vi "QuantelDataGrabSERI.vi"(9 "stop":bool) -> ()   [LabVIEW 2022 SP3]
uses:
  ScanningControl/Motion Controllers/-MotionRoutines/MotionGlobals.vi
  ScanningControl/Motion Controllers/NI_controller/-NI_MotionRoutines/MotionSys.ctl
  ScanningControl/-ScanSystem/Controls/location.ctl
  <instrlib>/Acqiris Bx/Acqiris Bx.lvlib
  <instrlib>/LeCroy Wave Series/LeCroy Wave Series.lvlib
  <vilib>/ptbypt/NI_PtbyPt.lvlib
  <vilib>/picture/picture.llb/imagedata.ctl
  <vilib>/Utility/miscctls.llb/LVRectTypeDef.ctl
  <vilib>/Utility/miscctls.llb/LVBoundsTypeDef.ctl
  <instrlib>/Acqiris Dx/Acqiris Dx.lvlib
  ScanningControl/Digitizers/-DigitizerRoutines/Digitizer.ctl
  ScanningControl/Motion Controllers/-MotionRoutines/ScanAxis.ctl
  ScanningControl/Motion Controllers/NI_controller/-NI_MotionRoutines/MotionParameters.ctl
  Patient Routines/PatientGlobals.vi
  ScanningControl/Digitizers/-DigitizerRoutines/DigitizerGlobals.vi
  ScanningControl/Motion Controllers/-MotionRoutines/3rdAxis.ctl
  <vilib>/DAQmx/write.llb/DAQmx Write (Digital Bool 1Line 1Point).vi
panel:
  in  "Overide Gain?":bool
  in  "Sector?":bool=TRUE
  in  "Fill\nSpace":bool
  out "File Name":string="none"
  in  "1:1\nAspect":bool
  out "append letter":i8=65
  in  "Visible":bool
  in  "Center":bool
  in  "c (m/s)":dbl=1485.0
  in  "Tab Control":enum32{"Acquire", "Custom Settings"}(tab)
  in  "Gain":dbl(ring)=0.2 items=["7"=8.0, "6"=4.0, "5"=2.0, "4"=0.8, "3"=0.4, "2"=0.2, "1"=0.08]
  in  "View Queue":bool
  out "No data\nEntering\nQueue":bool
  in  "Probe":u16(ring) items=["Aviso Sector 10 MHz", "Aviso Sector 20 MHz Retina", "Aviso Sector 20 MHz", "Aviso Lin50", "Custom"]
  out "fps":dbl format="%#.2g"
  in  "Save All Queue":bool
  in  "Flush Queue":bool
  in  "Pause":bool=TRUE
  out "In Queue":u8 max=50 step=1
  in  "Plane":i8(knob) min=0 max=12 step=3 scale=0.0..12.0
  in  "Patient Info":bool
  out "queue bar":u8(slide) scale=0.0..100.0
  in  "Scan Location":enum32{"Radio Selection 1", "Radio Selection 2"}(radio)
  in  "Save Raw":bool
  in  "SetDig":bool
  in  "Gate Length":dbl=0.15 format="%.6f"
  in  "LowTime":dbl=0.0001
  in  "Acquisition Parameters":T1={"Sampling Rate"=250.0, "Ref Delay (ms)"=0.0, "rf points per line"=2048, "rf lines"=256, "Dig Scale"=4.0} {"Dig Scale" items=["8 V"=8.0, "4 V"=4.0, "2 V"=2.0, "800 mV"=0.8, "400 mV"=0.4, "200 mV"=0.2, "80 mV"=0.08]; "rf lines" min=1; "rf points per line" min=1; "Ref Delay (ms)" format="%.2f"}
  in  "Filter Prams":T2={"low cutoff"=20, "order"=81, "high cutoff"=60}
  in  "Type of Mean":u16(ring)=4 items=["Mean from lines", "Mean just lines", "Poly Mean", "No mean", "Filter"]
  in  "distance?":bool=TRUE
  in  "Scan Info":T3
  in  "Timeout (s)":dbl=0.05
  in  "Software Gate":bool=TRUE
  in  "Bang Trig":bool=TRUE
  in  "N to save":u8=100 min=1 max=100 step=1
  out "Current Image":i32
  in  "Save Setting Profile":bool=TRUE
  in  "dB Range":cluster{i32, i32}(slide)={-65, 0}
  out "Raw data":dbl[][](graph)
  # "dB"
  # "Ruler"
  # "Do not adjust!!!!!"
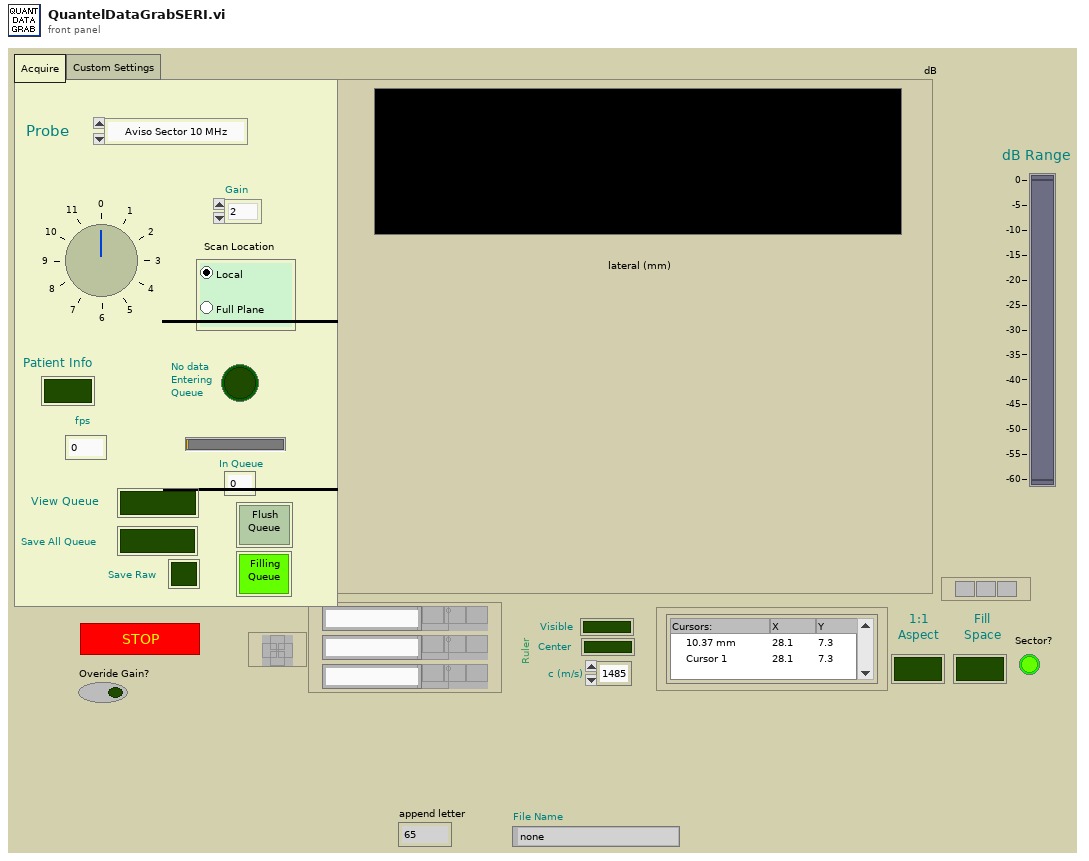
[diagram p1: front panel]
types:
  T1 = cluster{"Sampling Rate":dbl, "Ref Delay (ms)":dbl, "rf points per line":i32, "rf lines":i32, "Dig Scale":dbl}
  T2 = cluster{"low cutoff":i32, "order":i32, "high cutoff":i32}
  T3 = cluster{"delay":sgl, "pivot distance":sgl, "sector scan angle":sgl, "operator":string, "Scan Mode":string, "location":string}
  T4 = typedef "MotionParameters.ctl" = cluster{"No Motion?":bool, "Motion System":T5, "Motion Bd ID":u8, "Motion Profile":string, "# Axis":i8, "Reverse Z axis?":bool, "SMAC Axis":u16, "scan pair":T6, "RT fps":sgl, "Steps per mm":i32[], "Motor Parameters":cluster{"velocity ct/s":dbl[], "accel ct/s^2":dbl[]}, "One Way Scan":bool, "Reverse One Way Scan":bool, "Global Position (mm)":dbl[], "Plane":i32, "Distance between\nscan lines (um)":sgl, "Distance between\nscan planes (um)":sgl, "number of scan planes":i32, "Total steps in line":i32, "Xtra plane\ndistance  (um)":i32, "Xtra planes ":i32, "Add Axis":bool, "overshoot cts":i32, "BKPT Shift":i32, "Scan Start Time (ms)":u32, "ESP VISA":refnum<visa-resource-name>, "3rd Axis":T7, "GL Ref Out":refnum<k7>, "Galil Address":string}
  T5 = typedef "MotionSys.ctl" = enum16{"MM3000", "NI 735x", "Newport ESP", "No Motion Card", "Galil"}
  T6 = typedef "ScanAxis.ctl" = enum16{"y-(x) scan", "x-(y) scan", "z-(x) scan", "z-(y) scan", "y-(z) scan", "x-(z) scan", "w-(x) scan", "w-(y) scan", "w-(z) scan", "x-(w) scan", "y-(w) scan", "z-(w) scan"}
  T7 = typedef "3rdAxis.ctl" = u16
  T8 = typedef "LVBoundsTypeDef.ctl" = cluster{"Width":u32, "Height":u32}
  T9 = typedef "LVRectTypeDef.ctl" = cluster{"Left":i16, "Top":i16, "Right":i16, "Bottom":i16}
  T10 = typedef "Digitizer.ctl" = enum16{"Acqiris Digitizer", "NI Digitizer", "LeCroy", "GaGe", "AlazarTech", "No Digitizer", "Teledyne"}
  T11 = cluster{"gain":dbl, bool, "wfm":i16[][], "max queue size (-1, unlimited)":i32, bool}
  T12 = cluster{"DataBufferQ":refnum<queue>, "LastNQ":refnum<queue>, "LastN_JPG_Q":refnum<queue>, "Stop":refnum<notifier>}
  T13 = typedef "imagedata.ctl" = cluster{"image type":i32, "image depth":i32, "image":u8[], "mask":u8[], "colors":u32[], "Rectangle":cluster{"left":i16, "top":i16, "right":i16, "bottom":i16}}
  T14 = typedef "location.ctl" = enum16{"Automatic", "WCM Main", "Hawaii", "Columbia MM3000", "Columbia  NI System", "NYU", "RRI 2", "UHI Allen", "CUMC RT", "Chiba", "Stony Brook", "WCM Microscopy", "WCM Aeoretch", "WCM Optics Lab", "WCM Main 2Axis", "WCM Rotation", "WCM SAM SMAC", "SERI GP"}
  T15 = cluster{"Voltage Scale":dbl, "Offset":dbl, "Coupling":u16}
  T16 = cluster{"Source":u16, "Coupling":u16, "Slope":u16, "Level":dbl}
  T17 = cluster{"Source":u16, "Coupling":u16, "Slope":u16, "Level (mV)":dbl}
  T18 = cluster{"DataBufferQ":refnum<queue>, "LastNQ":refnum<queue>, "LastNBMPQ":refnum<queue>, "SaveRawN":refnum<notifier>, "StopN":refnum<notifier>}
  T19 = cluster{"NI Dig":refnum<k15>, "Lecroy":refnum<visa-resource-name>, "Alazar":i32, "Acqiris":string}
  T20 = typedef "DigitizerSettings.ctl" = cluster{"Digitizer delay (us) ":dbl, "rf points per line":i32, "lines per plane":i32, "Samp Rate (Hz)":dbl, "Additional dig delay (us)":dbl, "Voltage Scale":dbl, "Pre-Looks":i32, "Offset delay (us)":dbl, "bits A/D":i8, "Avg Num":i32, "DigTimeOut":sgl, "Rel Dig Delay":sgl, "Dig Ch":i32, "LeCroyCluster":cluster{"LeCroy Channels":bool[], "LC read pt offset":dbl, "Sweep Avg":bool}, "Main Digitizer":T10, "Dig Config":T21, "Digitizer ID Cluster":T22, "Trigger Settings":cluster{"Trig Source":u16, "Trig Coupling":u16, "Trig Slope":u16, "Level (mV)":dbl}, "Bulk Acq":bool, "Bulk Start Indexes":i32[], "Data Ref RF":refnum<data-value>, "NI ID/Channel":cluster{"NI ID":refnum<k15>, "NI CH":i32}[], "Total Dig CH":i32, "Xtra Ann Trig delay (us)":dbl, "Fix Z Delay?":bool, "One Way Transmission?":bool, "Data Ref Log":refnum<data-value>}
  T21 = typedef "DigConfig.ctl" = enum16{"Single channel", "2 Chans w/ 2 Acqiris", "2 Chans w/ 1 Acqiris", "5-CH Pulser New", "5-CH pulser w/ ann array", "5-pass style ann array", "Empty"}
  T22 = typedef "DigitizerID.ctl" = cluster{"Acqiris/Alazar/SP ID":u32[], "NI Instr Handles":refnum<k15>[], "LeCroy VISA":refnum<visa-resource-name>, "GaGe Handle":cluster{"Handle":u32, "Sample size":u32, "Resolution":i32, "Offset":i32, "Channels":u32, "Boards":u32}, "ATS Ref":string, "Acqiris Address":string[], "ADQRef":refnum<k24>, "adq_cu_ptr":refnum<k24>}
  T23 = cluster{"Handle":u32, "Sample size":u32, "Resolution":i32, "Offset":i32, "Channels":u32, "Boards":u32}
  T24 = typedef "LVStringsAndValuesArrayTypeDef_DBL.ctl" = cluster{"String":string, "Value":dbl}[]
  T25 = cluster{"Case name":string, "Distance between\nscan lines (mm)":sgl, "Acquistion Parameters":cluster{"Sampling Rate":dbl, "Ref Delay (ms)":dbl, "rf points per line":i32, "rf lines":i32, "Dig Scale":dbl}, "Timeout (s)":dbl, "Sector?":bool, "Filter Prams":cluster{"low cutoff":i32, "order":i32, "high cutoff":i32}, "Scan Info":cluster{"delay":sgl, "pivot distance":sgl, "sector scan angle":sgl, "operator":string, "Scan Mode":string, "location":string}}[]
  T26 = cluster{"Case name":string, "Distance between\nscan lines (mm)":sgl, "Acquistion Parameters":cluster{"Sampling Rate":dbl, "Ref Delay (ms)":dbl, "rf points per line":i32, "rf lines":i32, "Dig Scale":dbl}, "Timeout (s)":dbl, "Sector?":bool, "Filter Prams":cluster{"low cutoff":i32, "order":i32, "high cutoff":i32}, "Scan Info":cluster{"delay":sgl, "pivot distance":sgl, "sector scan angle":sgl, "operator":string, "Scan Mode":string, "location":string}}
  T27 = cluster{"Y Scale Offset":dbl, "Y Scale Multi":dbl, "X Scale Offset":dbl, "X Scale Multi":dbl, "Gate Distance":dbl}
  T28 = cluster{"data value reference":refnum<data-value>, "bytes to transfer":u32, "rf pts actual":u32}
  T29 = cluster{"Axis scaling Params":cluster{"X right":dbl, "X left":dbl, "Y low":dbl, "Y high":dbl}, "x scaled":dbl[][], "y scaled":dbl[][], "scales":cluster{"inc x (mm)":dbl, "inc y (mm)":dbl}, "Array":dbl[][], "pixels in x":i16, "pixels in y":i16}
  T30 = typedef "PatientInfoDef.ctl" = cluster{"Eye Selector":enum32{"Left", "Right"}, "Plane":i8, "First Name":string, "Last Name":string, "Notes":string, "Patient ID":string, "Scan Location":enum32{"Radio Selection 1", "Radio Selection 2"}}
  T31 = typedef "LVRangeTypeDef.ctl" = cluster{"Minimum":dbl, "Maximum":dbl, "Increment":dbl, "Minor Increment":dbl, "Start":dbl}
  T32 = typedef "LVPointDoubleTypeDef.ctl" = cluster{"Cursor X":dbl, "Cursor Y":dbl}
  T33 = cluster{"New Case Name":string, "Distance between\nscan lines (um)":sgl, "Acquisition Parameters":cluster{"Sampling Rate":dbl, "Ref Delay (ms)":dbl, "rf points per line":i32, "rf lines":i32, "Dig Scale":dbl}, "Timeout (s)":dbl, "Sector?":bool, "Filter Prams":cluster{"low cutoff":i32, "order":i32, "high cutoff":i32}, "Scan Info":cluster{"delay":sgl, "pivot distance":sgl, "sector scan angle":sgl, "operator":string, "Scan Mode":string, "location":string}}
  T34 = cluster{"gain":dbl, "status":bool, "Array":i16[][], "timeout in ms (-1)":i32, "status":bool}
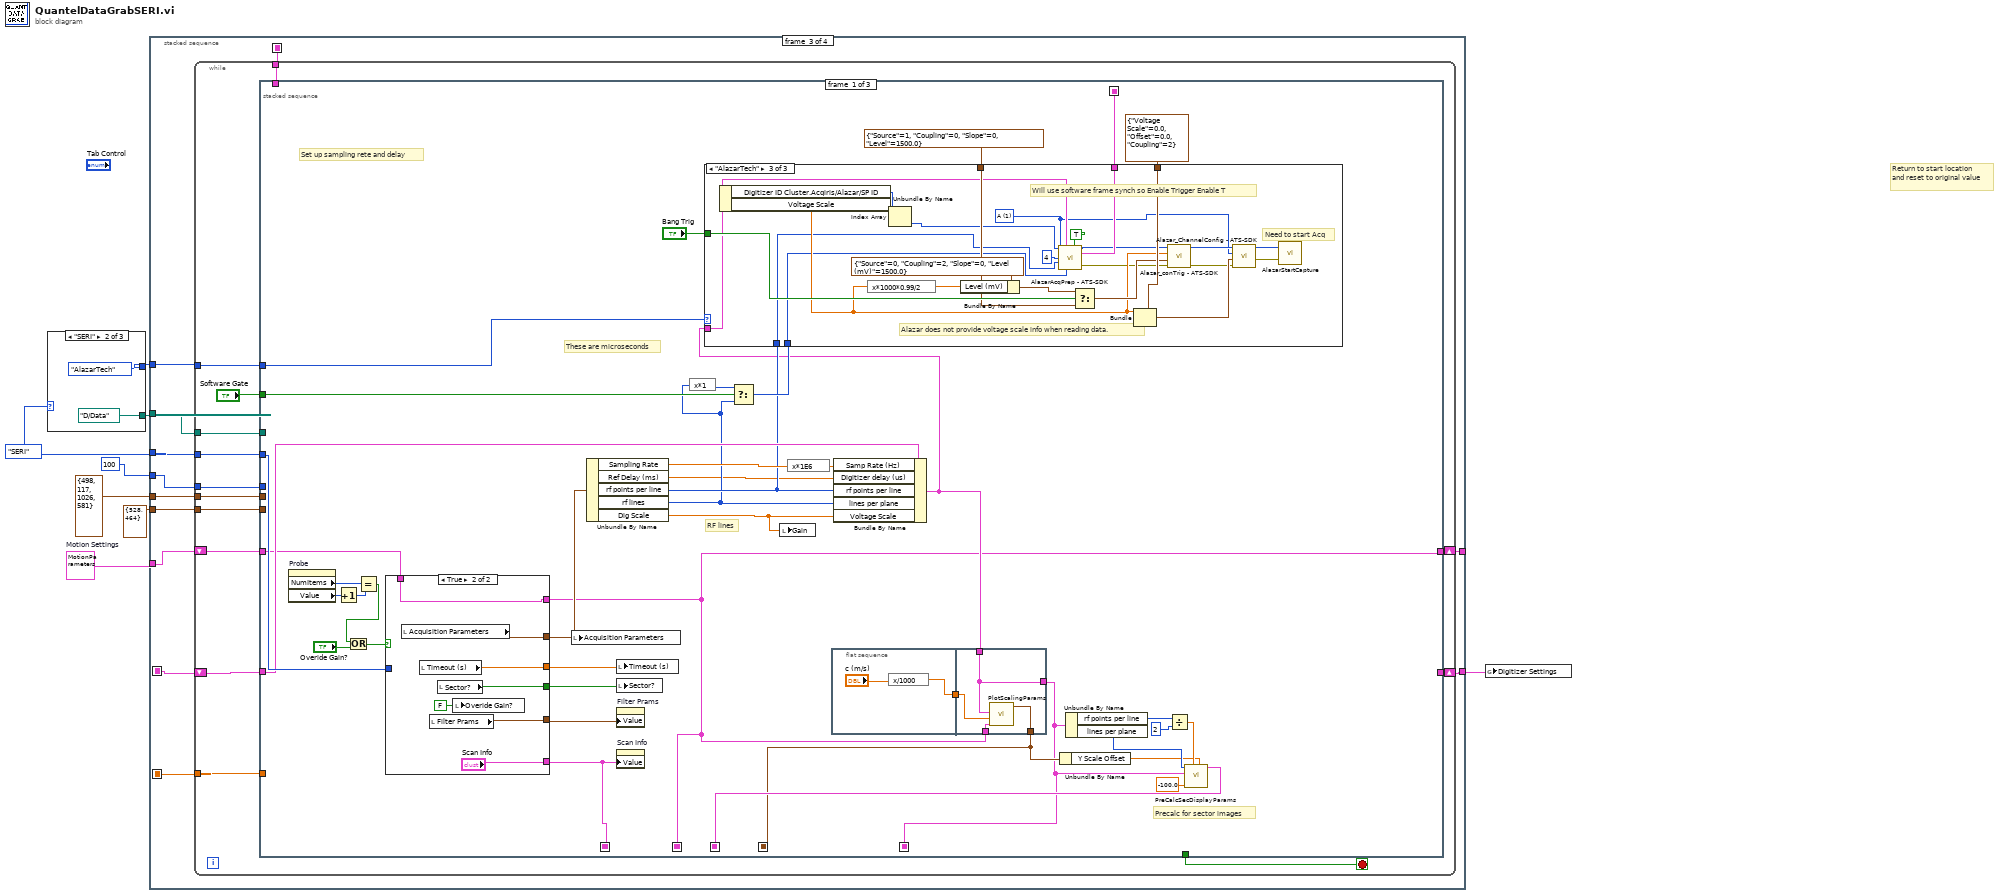
[diagram p0: block diagram]
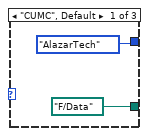
[diagram p2: hidden frame]
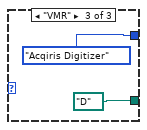
[diagram p3: hidden frame]
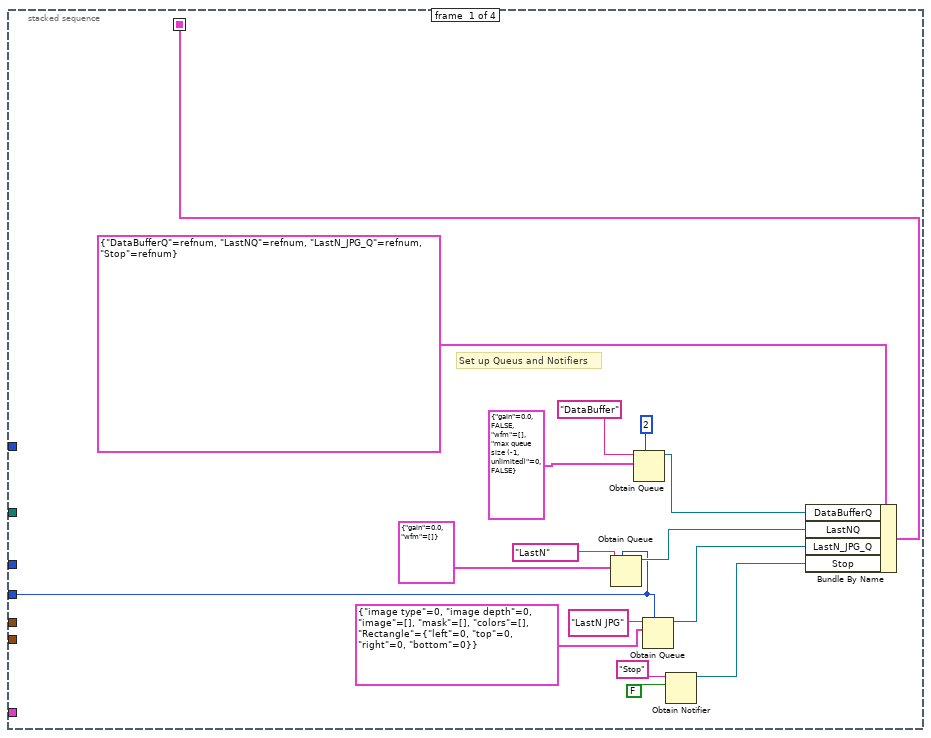
[diagram p4: hidden frame]
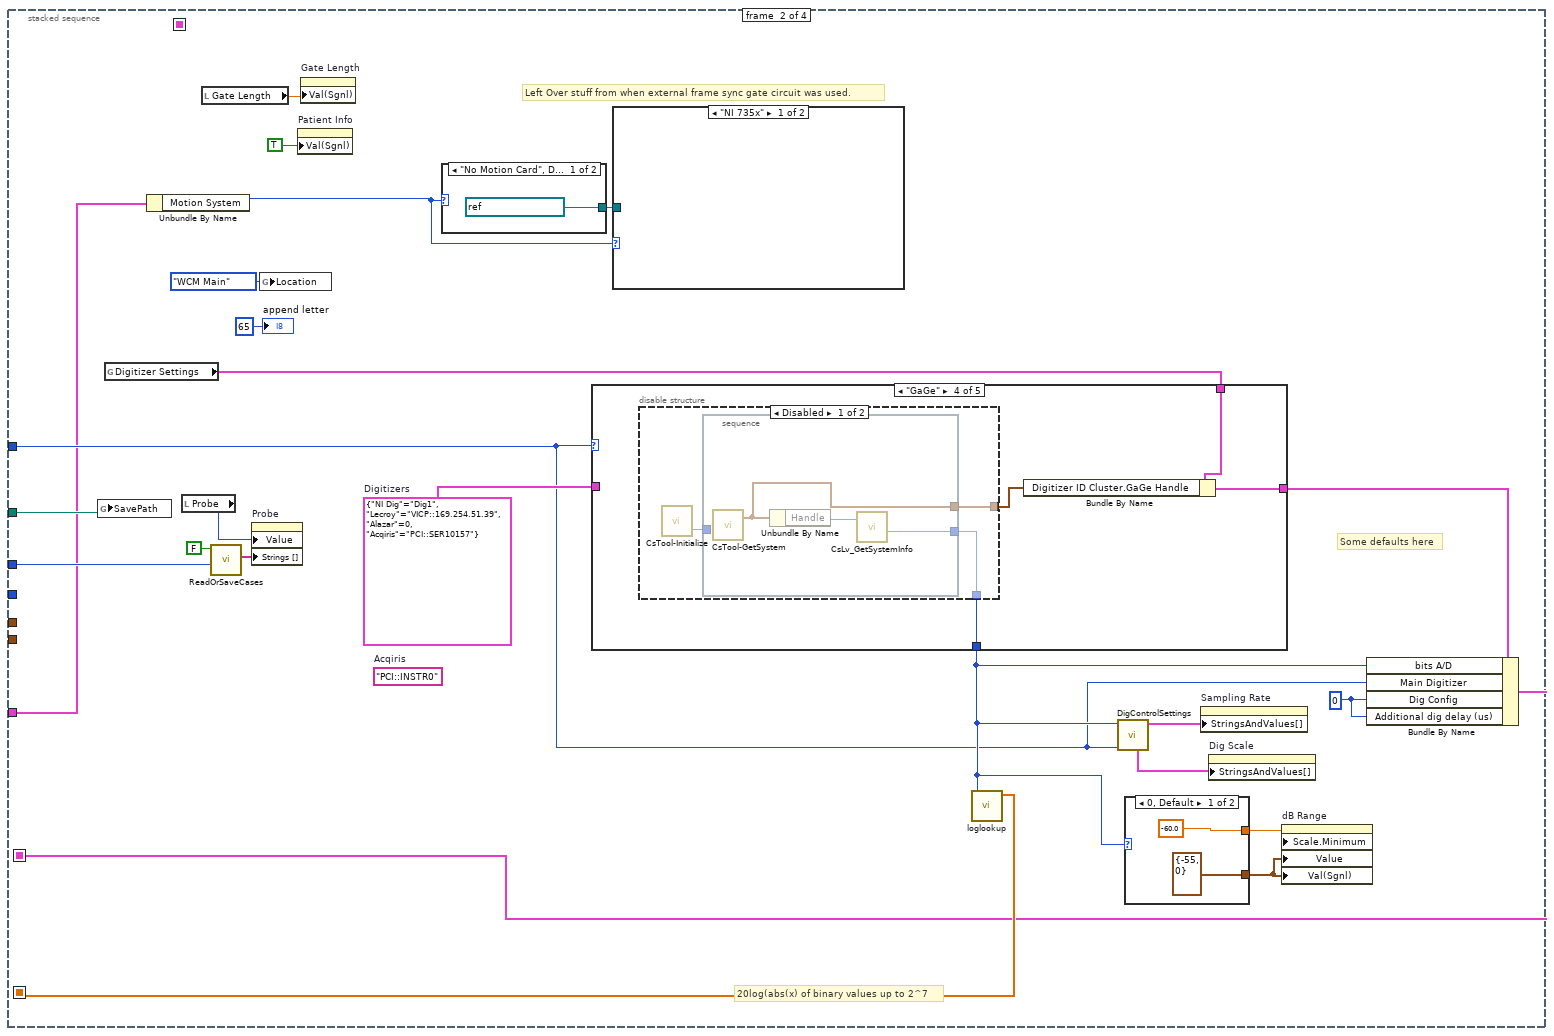
[diagram p5: hidden frame]
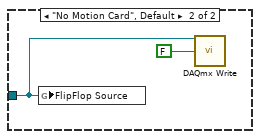
[diagram p6: hidden frame]
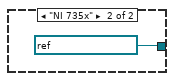
[diagram p7: hidden frame]
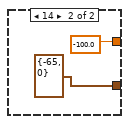
[diagram p8: hidden frame]
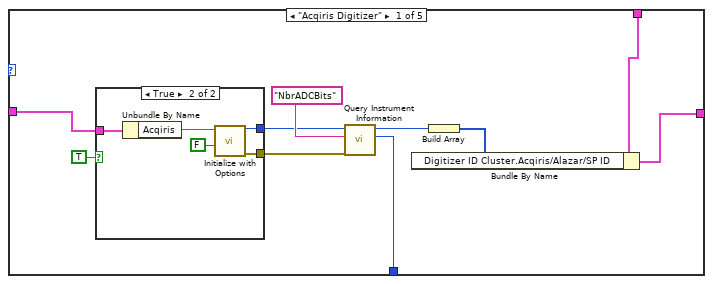
[diagram p9: hidden frame]
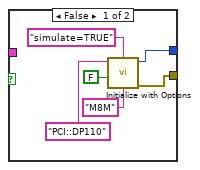
[diagram p10: hidden frame]
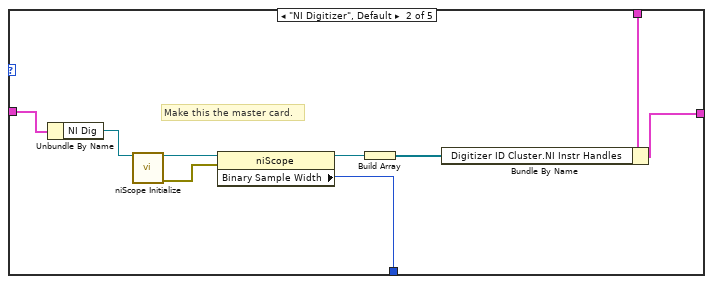
[diagram p11: hidden frame]
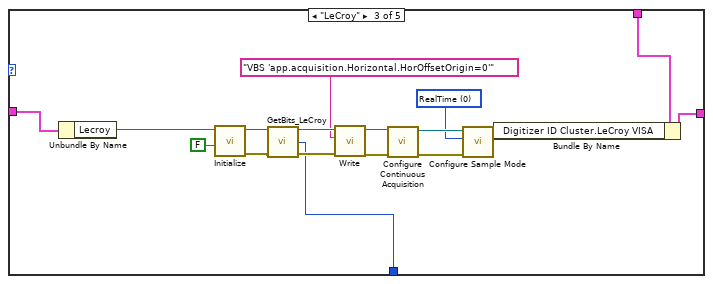
[diagram p12: hidden frame]
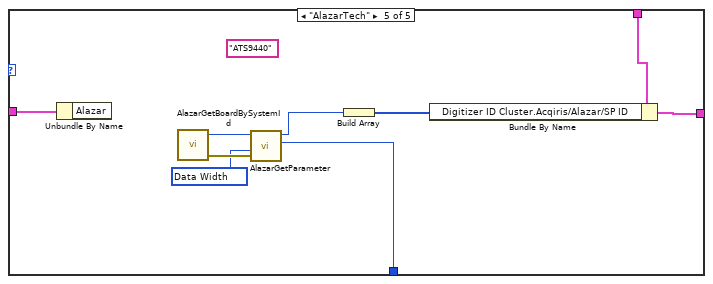
[diagram p14: hidden frame]
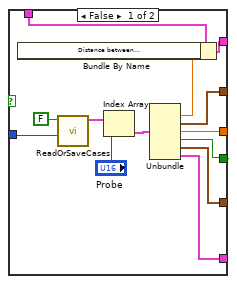
[diagram p15: hidden frame]
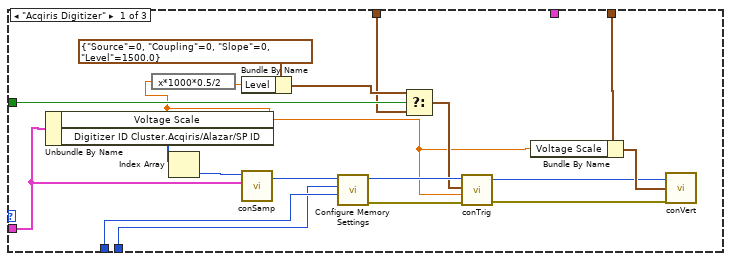
[diagram p16: hidden frame]
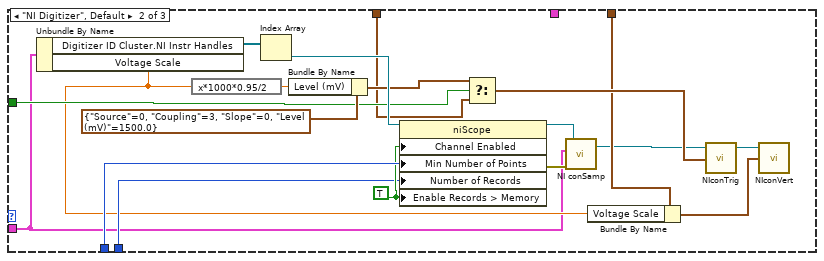
[diagram p17: hidden frame]
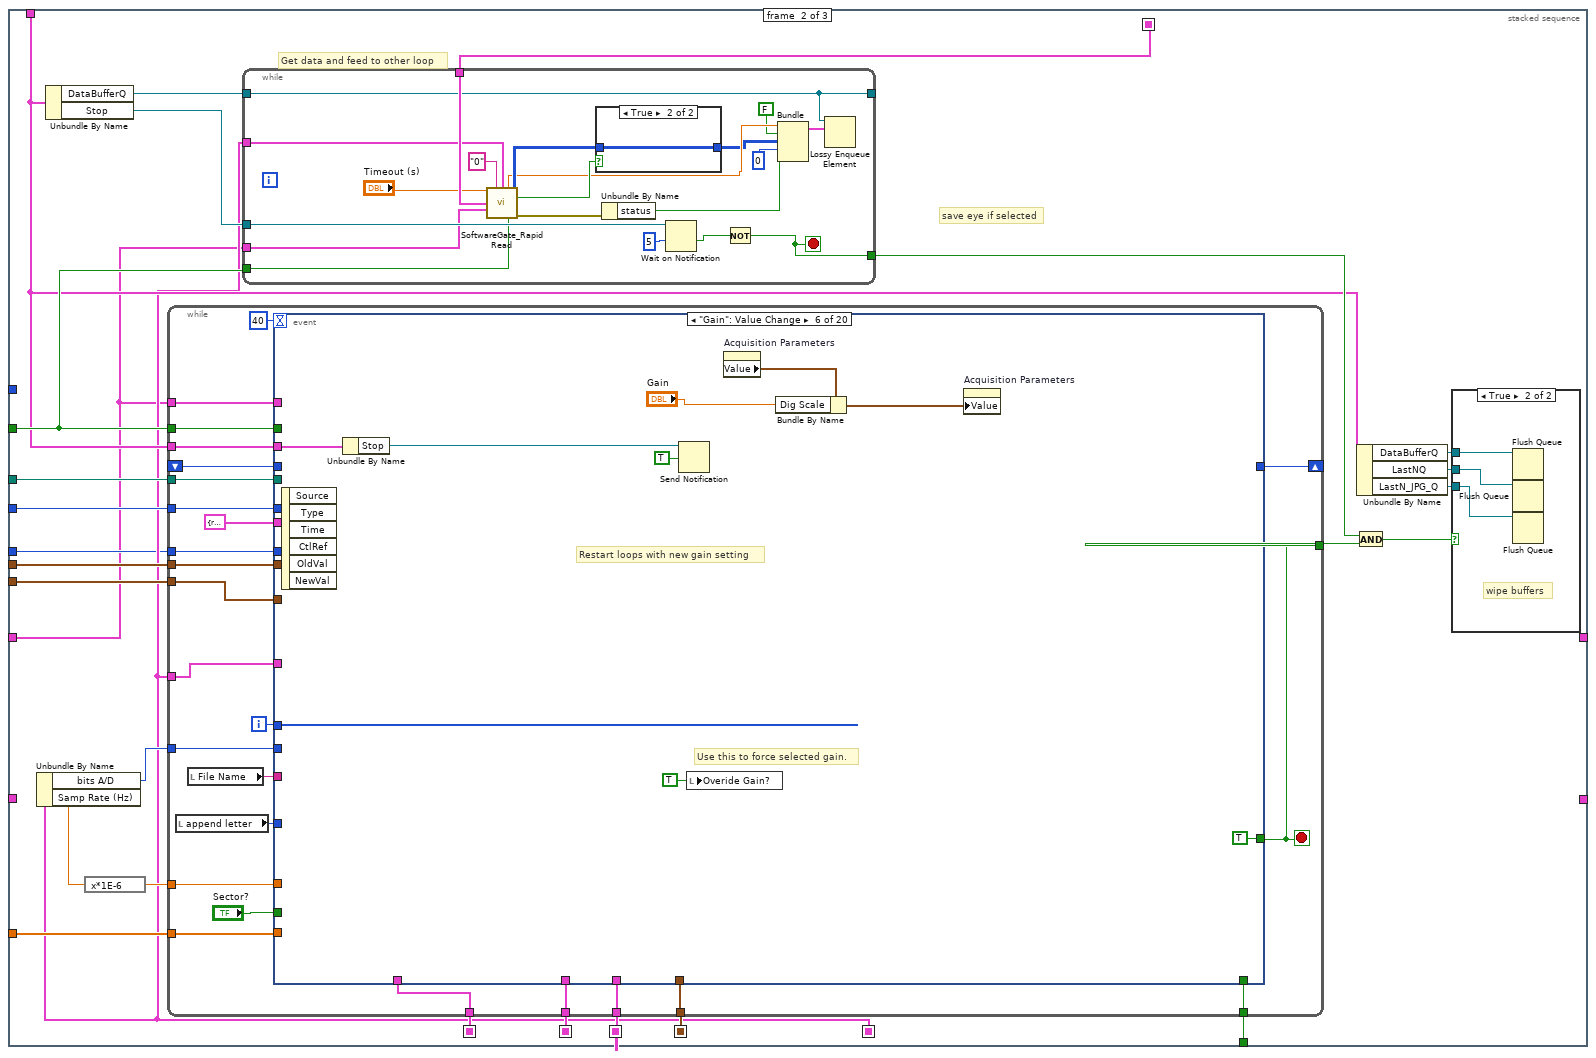
[diagram p18: hidden frame]
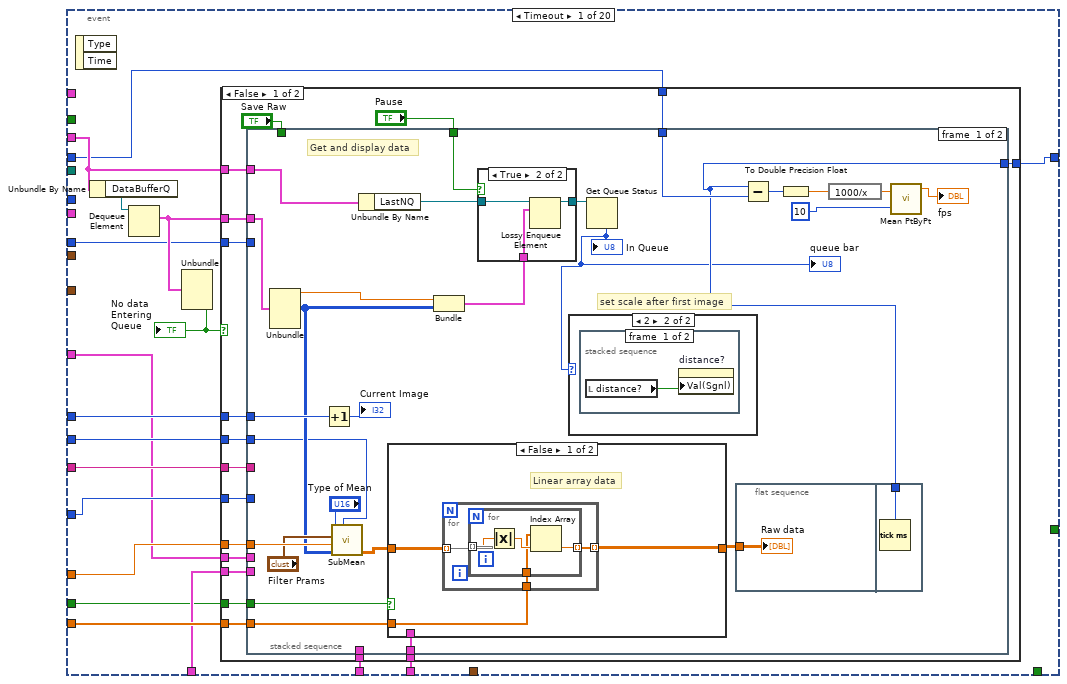
[diagram p20: hidden frame]
diagram:
  w3 = T4 {"No Motion?"=FALSE, "Motion System"=enum."No Motion Card", "Motion Bd ID"=1, "Motion Profile"="SMAC1", "# Axis"=1, "Reverse Z axis?"=TRUE, "SMAC Axis"=0, "scan pair"=enum."y-(x) scan", "RT fps"=6.0, "Steps per mm"=[1000, 1000, 1000, 1000], "Motor Parameters"={"velocity ct/s"=[10000.0, 10000.0, 10000.0, 50000.0], "accel ct/s^2"=[50000.0, 50000.0, 50000.0, 200000.0]}, "One Way Scan"=FALSE, "Reverse One Way Scan"=FALSE, "Global Position (mm)"=[], "Plane"=0, "Distance between\nscan lines (um)"=0.0, "Distance between\nscan planes (um)"=0.0, "number of scan planes"=1, "Total steps in line"=0, "Xtra plane\ndistance  (um)"=100, "Xtra planes "=1, "Add Axis"=FALSE, "overshoot cts"=200, "BKPT Shift"=0, "Scan Start Time (ms)"=0, "ESP VISA"="GPIB::1::INSTR", "3rd Axis"=1, "GL Ref Out"=refnum, "Galil Address"=""}  # Motion Settings
  w5 = enum16{"CUMC", "SERI", "VMR"}."SERI"
  # "Return to start location and reset to original value"
  n1 = case shown="\"SERI\"" w5 {
    tunnel: [path "F:/Data" ("SavePath") path "D:/Data" ("SavePath") path "D:/" ("SavePath")] -> w7
    tunnel: [Digitizer."AlazarTech" ("Main Digitizer") Digitizer."AlazarTech" ("Main Digitizer") Digitizer."Acqiris Digitizer" ("Main Digitizer")] -> w6
    frame "CUMC", Default {
    }
    frame "SERI" {
    }
    frame "VMR" {
    }
  }
  n2 = stacked-sequence {
    seq-local: [_ w54 _ _] -> [_ _ w140 _]
    seq-local: [w20 _ _ _] -> [_ _ w138 w701]
    seq-local: [_ w37 _ _] -> [_ _ w132 w702]
    tunnel: w6 -> [_ w36 w139 w708]
    tunnel: T8 {"Width"=528, "Height"=464} ("Plot Area:Size") -> [_ _ w137 _]
    tunnel: T9 {"Left"=498, "Top"=117, "Right"=1026, "Bottom"=581} ("Plot Area Bounds") -> [_ _ w136 _]
    tunnel: w7 -> [_ w45 w135 _]
    tunnel: w5 -> [_ w41 w134 _]
    tunnel: [_ _ w133 _] -> w2
    tunnel: w3 -> [_ w33 w131 _]
    tunnel: [_ _ w130 _] -> _
    tunnel: 100 ("max queue size (-1, unlimited)") -> [w15 _ w129 _]
    frame #0 {
      # "Set up Queus and Notifiers"
      n3 = Obtain Queue ("LastN")(max queue size (-1, unlimited)=w15, name (unnamed)="LastN", element data type=cluster{"gain":dbl, "wfm":i16[][]} {"gain"=0.0, "wfm"=[]}) -> (queue out=w19:refnum<queue>)  [unwired: 2 in, 2 out]
      n4 = Obtain Queue(max queue size (-1, unlimited)=2, name (unnamed)="DataBuffer", element data type=T11 {"gain"=0.0, FALSE, "wfm"=[], "max queue size (-1, unlimited)"=0, FALSE}) -> (queue out=w16:refnum<queue>)  [unwired: 2 in, 2 out]
      n5 = Obtain Queue ("LastNBMP")(max queue size (-1, unlimited)=w15, name (unnamed)="LastN JPG", element data type=T13 {"image type"=0, "image depth"=0, "image"=[], "mask"=[], "colors"=[], "Rectangle"={"left"=0, "top"=0, "right"=0, "bottom"=0}} ("Image Data")) -> (queue out=w25:refnum<queue>)  [unwired: 2 in, 2 out]
      n6 = Obtain Notifier ("Raw eye")(name (unnamed)="Stop", notification data type=FALSE) -> (notifier out=w21:refnum<notifier>)  [unwired: 2 in, 2 out]
      n7 = Bundle By Name(cluster=T12 {"DataBufferQ"=refnum, "LastNQ"=refnum, "LastN_JPG_Q"=refnum, "Stop"=refnum} ("Qs and Notis"), "DataBufferQ"=w16, "LastNQ"=w19, "LastN_JPG_Q"=w25, "Stop"=w21) -> (w20:T12)
    }
    frame #1 {
      (unwired) "PCI::INSTR0"  # Acqiris
      w51 = T19 {"NI Dig"="Dig1", "Lecroy"="VICP::169.254.51.39", "Alazar"=0, "Acqiris"="PCI::SER10157"}  # Digitizers
      w35 = 0 ("Dig Config")
      # "Left Over stuff from when external frame sync gate circuit was used."
      # "Some defaults here"
      # "20log(abs(x) of binary values up to 2^7"
      n8 = global write "MotionGlobals.vi" "SavePath"(w45) -> ()
      n9 = global read "DigitizerGlobals.vi" "Digitizer Settings"() -> (w34:T20)
      n10 = Unbundle By Name(w33) -> ("Motion System"=w32:T5)
      n11 = local read "Probe"() -> (w40:u16)
      n12 = local read "Gate Length"() -> (w53:dbl)
      n13 = call "ReadOrSaveCases.vi"("Location"=w41, "Save(T)\\Read(F)"=FALSE ("Save(T)\\Read(F)")) -> ("Case List"=w42:string[])  [unwired: 8 in, 1 out]
      n14 = property on="Probe" class="Ring (strict)"("Value"=w40, "Strings []"=w42) -> ()  [unwired: 2 in, 2 out]
      n15 = global write "MotionGlobals.vi" "Location"(location."WCM Main" ("Location")) -> ()
      n16 = property on="Patient Info" class="Bool (strict)"("Val(Sgnl)"=TRUE ("Value (Signaling)")) -> ()  [unwired: 2 in, 2 out]
      n17 = property on="Gate Length" class="DigNum (strict)"("Val(Sgnl)"=w53) -> ()  [unwired: 2 in, 2 out]
      n18 = case shown="\"No Motion Card\", Default" w32 {
        tunnel: [refnum<k21> "Dev1 FlipFlop" ("FlipFlop Source") refnum<k21> "QuantFlipFlop" ("FlipFlop Source")] -> w31
        frame "No Motion Card", Default {
        }
        frame "NI 735x" {
        }
      }
      n19 = case shown="\"GaGe\"" w36 {
        tunnel: [w71 w92 w94 w113 w120] -> w39
        tunnel: w51 -> [w70 w89 w98 _ w128]
        tunnel: [w67 w85 w95 w111 w126] -> w38
        tunnel: w34 -> [w63 w84 w93 w110 w125]
        frame "Acqiris Digitizer" {
          n20 = case shown="True" TRUE {
            tunnel: w70 -> [_ w82]
            tunnel: [w77 w81] -> w66
            tunnel: [w76 w80] -> w65
            frame False {
              n21 = call <instrlib>:"Initialize with Options.vi"("Options String (null string)"="simulate=TRUE", "Resource Name (PCI::INSTR0)"="PCI::DP110" ("Simulation Options (null string)"), "Simulation Options (null string)"="M8M" ("Options String (null string)"), "Reset (T: Reset)"=FALSE) -> ("Instrument ID"=w77:u32, "error out"=w76:errorcluster)  [unwired: 2 in, 2 out]
            }
            frame True {
              n22 = Unbundle By Name(w82) -> ("Acqiris"=w79:string)
              n23 = call <instrlib>:"Initialize with Options.vi"("Resource Name (PCI::INSTR0)"=w79, "Reset (T: Reset)"=FALSE) -> ("Instrument ID"=w81:u32, "error out"=w80:errorcluster)  [unwired: 4 in, 2 out]
            }
          }
          n24 = call <instrlib>:"Query Instrument Information.vi"("Instrument ID"=w66, "Parameter String"="NbrADCBits", "error in (no error)"=w65) -> ("dup Instrument ID"=w69:u32, "Info Value (I32)"=w71:i32)  [unwired: 1 in, 4 out]
          n25 = Build Array(w69) -> (w68:u32[])
          n26 = Bundle By Name(cluster=w63, "Digitizer ID Cluster.Acqiris/Alazar/SP ID"=w68) -> (w67:T20)
        }
        frame "NI Digitizer", Default {
          # "Make this the master card."
          n27 = Unbundle By Name(w89) -> ("NI Dig"=w88:refnum<k15>)
          n28 = call <instrlib>:"niScope Initialize.vi"("resource name"=w88) -> ("instrument handle"=w91:refnum<k15>, "error out"=w90:errorcluster)  [unwired: 3 in, 10 out]
          n29 = property class="niScope"(reference=w91, error in=w90) -> (reference out=w87:refnum<k15>, "Binary Sample Width"=w92:i32)  [unwired: 1 out]
          n30 = Build Array(w87) -> (w86:refnum<k15>[])
          n31 = Bundle By Name(cluster=w84, "Digitizer ID Cluster.NI Instr Handles"=w86) -> (w85:T20)
        }
        frame "LeCroy" {
          w104 = u16 0 items=["RealTime", "RIS", "Sequence", "Roll", "WaveStream"] ("Sample Mode (0: RealTime)")
          n32 = Unbundle By Name(w98) -> ("Lecroy"=w97:refnum<visa-resource-name>)
          n33 = call <instrlib>:"Initialize.vi"("Reset? (T: Yes)"=FALSE, "VISA resource name"=w97) -> ("error out"=w107:errorcluster, "VISA resource name out"=w108:refnum<visa-resource-name>)  [unwired: 8 in]
          n34 = call "GetBits_LeCroy.vi"("VISA resource name"=w108, "error in (no error)"=w107) -> ("VISA resource name out"=w100:refnum<visa-resource-name>, "Nom_Bits"=w94:i16, "error out"=w101:errorcluster)  [unwired: 11 in]
          n35 = call <instrlib>:"Write.vi"("error in (no error)"=w101, "Write Buffer"="VBS 'app.acquisition.Horizontal.HorOffsetOrigin=0'", "VISA resource name"=w100) -> ("error out"=w102:errorcluster, "VISA resource name out"=w103:refnum<visa-resource-name>)  [unwired: 6 in, 1 out]
          n36 = call <instrlib>:"Configure Continuous Acquisition.vi"("error in (no error)"=w102, "VISA resource name"=w103) -> ("error out"=w106:errorcluster, "VISA resource name out"=w105:refnum<visa-resource-name>)  [unwired: 8 in]
          n37 = call <instrlib>:"Configure Sample Mode.vi"("error in (no error)"=w106, "Sample Mode (0: RealTime)"=w104, "VISA resource name"=w105) -> ("VISA resource name out"=w96:refnum<visa-resource-name>)  [unwired: 7 in, 1 out]
          n38 = Bundle By Name(cluster=w93, "Digitizer ID Cluster.LeCroy VISA"=w96) -> (w95:T20)
        }
        frame "GaGe" {
          n39 = disable-structure shown="Disabled" {
            disable-tunnel: [w116 _] -> w113
            disable-tunnel: [w114 _] -> w112
            frame Disabled {
              n40 = call <userlib>:"CsTool-Initialize.vi"() -> ("Error Code"=w115:i32)  [unwired: 1 out]
              n41 = stacked-sequence {
                tunnel: [w118] -> w116
                tunnel: w115 -> [_]
                tunnel: [w117] -> w114
                frame #0 {
                  n42 = call <userlib>:"CsTool-GetSystem.vi"() -> ("Handle Cluster"=w117:T23)  [unwired: 4 in, 1 out]
                  n43 = Unbundle By Name(w117) -> ("Handle"=w119:u32)
                  n44 = call <userlib>:"CsLv_GetSystemInfo.vi"("Handle"=w119) -> ("Sample Bits"=w118:u32)  [unwired: 6 out]
                }
              }
            }
            frame Enabled {
            }
          }
          n45 = Bundle By Name(cluster=w110, "Digitizer ID Cluster.GaGe Handle"=w112) -> (w111:T20)
        }
        frame "AlazarTech" {
          w122 = u32 268435465 items=["Data Width"=268435465, "Set/Get Async BuffSize"=268435513, "Set/Get Async Buffcount"=268435520, "Get Data Format"=268435522, "Get Samples Per Timestamp Clock"=268435524, "Get Records Captured"=268435525, "Get Async Buffers Pending"=268435536, "Get Async Buffers Pending Full"=268435537, "Get Async Buffers Pending Empty"=268435538, "ECC Mode"=268435528, "Get Aux Input Level"=268435529, "Get Channels Per Board"=268435568, "Pack Mode"=268435570, "Get FPGA Temperature"=268435584] ("Parameter")
          (unwired) "ATS9440" ("BoardToVerify")
          n46 = Unbundle By Name(w128) -> ()  [unwired: 1 out]
          n47 = call "AlazarGetBoardBySystemId.vi"() -> ("error out"=w123:errorcluster, "Handle"=w124:u64)  [unwired: 3 in, 1 out]
          n48 = call "AlazarGetParameter.vi"("error in (no error)"=w123, "Parameter"=w122, "Handle"=w124) -> ("Value"=w120:i32, "Handle"=w121:u64)  [unwired: 1 in, 2 out]
          n49 = Build Array(w121) -> (w127:u64[])
          n50 = Bundle By Name(cluster=w125, "Digitizer ID Cluster.Acqiris/Alazar/SP ID"=w127) -> (w126:T20)
        }
      }
      n51 = case shown="\"NI 735x\"" w32 {
        tunnel: w31 -> [_ w55]
        frame "NI 735x" {
        }
        frame "No Motion Card", Default {
          n52 = global write "MotionGlobals.vi" "FlipFlop Source"(w55) -> ()
          n53 = call-poly <vilib>:"DAQmx Write.vi"("task/channels in"=w55, "data"=FALSE) -> ()  [unwired: 11 in, 3 out]
        }
      }
      n54 = call "loglookup.vi"("A/D bits"=w39) -> ("Log Lookup"=w54:sgl[])  [unwired: 2 in, 3 out]
      n55 = call "DigControlSettings.vi"(8:w36, 11:w39) -> ("Sampling Rates"=w48:T24, "Voltage Scale"=w47:T24)  [unwired: 5 in, 3 out]
      n56 = case shown="0, Default" w39 {
        tunnel: [-60.0 ("Scale.Range:Maximum") -100.0 ("Scale.Range:Maximum")] -> w46
        tunnel: [cluster{i32, i32} {-55, 0} ("dB Range") cluster{i32, i32} {-65, 0} ("dB Range")] -> w44
        frame 0, Default {
        }
        frame 14 {
        }
      }
      n57 = property on="Sampling Rate" class="Ring (strict)"("StringsAndValues[]"=w48) -> ()  [unwired: 2 in, 2 out]
      n58 = property on="Dig Scale" class="Ring (strict)"("StringsAndValues[]"=w47) -> ()  [unwired: 2 in, 2 out]
      n59 = property on="dB Range" class="Slide (strict)"("Scale.Minimum"=w46, "Value"=w44, "Val(Sgnl)"=w44) -> ()  [unwired: 2 in, 2 out]
      n60 = Bundle By Name(cluster=w38, "bits A/D"=w39, "Main Digitizer"=w36, "Dig Config"=w35, "Additional dig delay (us)"=w35) -> (w37:T20)
      "append letter" <- i8 65 ("append letter")
    }
    frame #2 {
      n61 = while {
        tunnel: w140 -> [w154]
        tunnel: w139 -> [w152]
        tunnel: w138 -> [w147]
        tunnel: w137 -> [w151]
        tunnel: w136 -> [w150]
        tunnel: w135 -> [w148]
        tunnel: w134 -> [w146]
        shift-right: [w144] -> w133
        shift-left: w132 -> [w145]
        shift-right: [w142] -> w130
        shift-left: w131 -> [w143]
        tunnel: w129 -> [w141]
        stop <- w153 stop-if-true
        n62 = stacked-sequence {
          seq-local: [w164 _ _] -> [_ w304 _]
          seq-local: [w172 _ _] -> [_ w303 _]
          seq-local: [w193 _ _] -> [_ w297 w692]
          seq-local: [w188 _ _] -> [_ w296 _]
          seq-local: [w161 _ _] -> [_ w285 w690]
          seq-local: [w159 _ _] -> [_ w286 _]
          tunnel: w154 -> [_ w306 _]
          tunnel: [_ w305 _] -> w153
          tunnel: w152 -> [w183 _ w691]
          tunnel: w147 -> [_ w287 _]
          tunnel: w151 -> [_ w299 _]
          tunnel: w150 -> [_ w298 _]
          tunnel: "Software Gate" -> [w189 w295 _]
          tunnel: w148 -> [_ w294 _]
          tunnel: w146 -> [w179 w293 _]
          tunnel: w145 -> [w175 _ _]
          tunnel: [_ _ w690] -> w144
          tunnel: w143 -> [w160 w283 _]
          tunnel: [w159 _ _] -> w142
          tunnel: w141 -> [_ w284 _]
          frame #0 {
            # "Precalc for sector images"
            # "RF lines"
            # "Set up sampling rete and delay"
            # "These are microseconds"
            n63 = property on="Probe" class="Ring (strict)"() -> ("NumItems"=w181:u32, "Value"=w182:u16)  [unwired: 2 in, 2 out]
            n64 = Increment(x=w182) -> (x+1=w180:u16)
            n65 = Equal?(x=w181, y=w180) -> (x = y?=w157:bool)
            n66 = Or(x=w157, y="Overide Gain?") -> (x .or. y?=w156:bool)
            n67 = case shown="True" w156 {
              tunnel: [w204 w220] -> w178
              tunnel: [w207 w219] -> w192
              tunnel: [w208 "Scan Info"] -> w188
              tunnel: [w205 w217] -> w185
              tunnel: [w206 w215] -> w184
              tunnel: w179 -> [w209 _]
              tunnel: w160 -> [w203 w216]
              tunnel: [w201 w216] -> w159
              frame False {
                n68 = call "ReadOrSaveCases.vi"("Location"=w209, "Save(T)\\Read(F)"=FALSE ("Save(T)\\Read(F)")) -> ("CaseArray"=w212:T25)  [unwired: 8 in, 1 out]
                n69 = Index Array(array=w212, index="Probe") -> (element=w211:T26)
                n70 = Unbundle(w211) -> ("Distance between\nscan lines (mm)"=w202:sgl, "Acquistion Parameters"=w204:T1, "Timeout (s)"=w205:dbl, "Sector?"=w206:bool, "Filter Prams"=w207:T2, "Scan Info"=w208:T3)  [unwired: 1 out]
                n71 = Bundle By Name(cluster=w203, "Distance between\nscan lines (um)"=w202) -> (w201:T4)
              }
              frame True {
                n72 = local read "Acquisition Parameters"() -> (w220:T1)
                n73 = local read "Timeout (s)"() -> (w217:dbl)
                n74 = local read "Filter Prams"() -> (w219:T2)
                n75 = local read "Sector?"() -> (w215:bool)
                n76 = local write "Overide Gain?"(FALSE ("Overide Gain?")) -> ()
              }
            }
            n77 = local write "Acquisition Parameters"(w178) -> ()
            n78 = Unbundle By Name(w178) -> ("Sampling Rate"=w194:dbl, "Ref Delay (ms)"=w169:dbl, "rf points per line"=w174:i32, "rf lines"=w171:i32, "Dig Scale"=w158:dbl)
            n79 = local write "Timeout (s)"(w185) -> ()
            n80 = local write "Sector?"(w184) -> ()
            n81 = property on="Filter Prams" class="Clust (strict)"("Value"=w192) -> ()  [unwired: 2 in, 2 out]
            n82 = property on="Scan Info" class="Clust (strict)"("Value"=w188) -> ()  [unwired: 2 in, 2 out]
            n83 = expression code="x*1"(w171) -> (w191:i32)
            n84 = Select(t=w191, s=w189, f=w171) -> (s? t:f=w190:i32)
            n85 = local write "Gain"(w158) -> ()
            n86 = expression code="x*1E6"(w194) -> (w168:dbl)
            n87 = flat-sequence {
              tunnel: [w195] -> w163
              tunnel: w162 -> [w199]
              tunnel: [w200] -> w164
              tunnel: w163 -> [w198]
              tunnel: [w199] -> w161
              tunnel: w159 -> [w197]
              frame #0 {
                n88 = expression code="x/1000"("c (m/s)") -> (w195:dbl)
              }
              frame #1 {
                n89 = call "PlotScalingParams.vi"("Motion Settings In"=w197, "c mm/mics"=w198, "Digitizer Settings"=w199) -> ("Cluster"=w200:T27)  [unwired: 6 in, 2 out]
              }
            }
            n90 = Bundle By Name(cluster=w175, "Samp Rate (Hz)"=w168, "Digitizer delay (us)"=w169, "rf points per line"=w174, "lines per plane"=w171, "Voltage Scale"=w158) -> (w162:T20)
            n91 = case shown="\"AlazarTech\"" w183 {
              tunnel: w174 -> [w236 w258 w262]
              tunnel: w190 -> [w235 w253 w263]
              tunnel: [_ _ w267] -> w193
              tunnel: "Bang Trig" -> [w225 w249 w280]
              tunnel: T16 {"Source"=1, "Coupling"=0, "Slope"=0, "Level"=1500.0} ("Trigger") -> [w224 w246 w279]
              tunnel: T15 {"Voltage Scale"=0.0, "Offset"=0.0, "Coupling"=2} ("V scale") -> [w223 w245 w276]
              tunnel: w162 -> [w222 w240 w266]
              frame "Acqiris Digitizer" {
                n92 = Unbundle By Name(w222) -> ("Voltage Scale"=w221:dbl, "Digitizer ID Cluster.Acqiris/Alazar/SP ID"=w239:u32[])
                n93 = expression code="x*1000*0.5/2"(w221) -> (w228:dbl)
                n94 = Index Array(array=w239) -> (element=w238:u32)  [unwired: 1 in]
                n95 = Bundle By Name(cluster=T16 {"Source"=0, "Coupling"=0, "Slope"=0, "Level"=1500.0} ("Trigger"), "Level"=w228) -> (w226:T16)
                n96 = call "conSamp.vi"("Digitizer Settings"=w222, "InstrumentID"=w238) -> ("DUP ID"=w237:u32)  [unwired: 2 in, 1 out]
                n97 = call <instrlib>:"Configure Memory Settings.vi"("Number of Samples (1000)"=w236, "Number of Segments (1)"=w235, "Instrument ID"=w237) -> ("error out"=w231:errorcluster, "dup Instrument ID"=w233:u32)  [unwired: 1 in, 2 out]
                n98 = Select(t=w226, s=w225, f=w224) -> (s? t:f=w227:T16)
                n99 = call "conTrig.vi"("error in"=w231, "Voltage Scale"=w221, "Trigger"=w227, "InstrumentID"=w233) -> ("error out"=w230:errorcluster, "dup id"=w232:u32)  [unwired: 1 in]
                n100 = Bundle By Name(cluster=w223, "Voltage Scale"=w221) -> (w234:T15)
                n101 = call "conVert.vi"("InstrumentID"=w232, "V scale"=w234, "error in"=w230) -> ()  [unwired: 3 in, 2 out]
              }
              frame "NI Digitizer", Default {
                w255 = TRUE
                n102 = Unbundle By Name(w240) -> ("Digitizer ID Cluster.NI Instr Handles"=w254:refnum<k15>[], "Voltage Scale"=w242:dbl)
                n103 = expression code="x*1000*0.95/2"(w242) -> (w250:dbl)
                n104 = Index Array(array=w254) -> (element=w251:refnum<k15>)  [unwired: 1 in]
                n105 = Bundle By Name(cluster=T17 {"Source"=0, "Coupling"=3, "Slope"=0, "Level (mV)"=1500.0} ("Trigger Settings"), "Level (mV)"=w250) -> (w248:T17)
                n106 = property class="niScope"(reference=w251, "Channel Enabled"=w255, "Min Number of Points"=w258, "Number of Records"=w253, "Enable Records > Memory"=w255) -> (reference out=w257:refnum<k15>, error out=w256:errorcluster)  [unwired: 1 in]
                n107 = Select(t=w248, s=w249, f=w246) -> (s? t:f=w247:T16)
                n108 = call "NI conSamp.vi"("error in"=w256, "Digitizer Settings"=w240, "InstrumentID"=w257) -> ("DUP ID"=w241:refnum<k15>)  [unwired: 1 in, 1 out]
                n109 = Bundle By Name(cluster=w245, "Voltage Scale"=w242) -> (w244:T15)
                n110 = call "NIconTrig.vi"("Trigger"=w247, "InstrumentID"=w241) -> ("dup id"=w243:refnum<k15>)  [unwired: 1 in, 2 out]
                n111 = call "NIconVert.vi"("InstrumentID"=w243, "V scale"=w244) -> ()  [unwired: 2 in, 4 out]
              }
              frame "AlazarTech" {
                w260 = u32 1 items=["A"=1, "B"=2, "A + B"=3, "C"=4, "A + C"=5, "A + B"=6, "D"=8, "A + D"=9, "B + D"=10, "C + D"=12, "A + B + C + D"=15] ("Channel")
                # "Will use software frame synch so Enable Trigger Enable T"
                # "Need to start Acq"
                # "Alazar does not provide voltage scale info when reading data."
                n112 = Unbundle By Name(w266) -> ("Digitizer ID Cluster.Acqiris/Alazar/SP ID"=w282:u32[], "Voltage Scale"=w269:dbl)
                n113 = expression code="x*1000*0.99/2"(w269) -> (w281:dbl)
                n114 = Index Array(array=w282) -> (element=w261:u32)  [unwired: 1 in]
                n115 = Bundle By Name(cluster=T17 {"Source"=0, "Coupling"=2, "Slope"=0, "Level (mV)"=1500.0} ("Trigger Settings"), "Level (mV)"=w281) -> (w277:T17)
                n116 = call "AlazarAcqPrep - ATS-SDK.vi"("Handle"=w261, "Digitizer Settings"=w266, "Enable Trigger Enable"=TRUE, "Channel"=w260, "BuffCount"=4, "rf points per line"=w262, "rf lines per buffer"=w263) -> ("Handle Out"=w259:u32, "AlazarCluster"=w267:T28, "error out"=w268:errorcluster)  [unwired: 5 in, 1 out]
                n117 = Select(t=w277, s=w280, f=w279) -> (s? t:f=w270:T16)
                n118 = Bundle(cluster=w276, "Voltage Scale"=w269) -> (w273:T15)  [unwired: 2 in]
                n119 = call "Alazar_conTrig - ATS-SDK.vi"("error in (no error)"=w268, "Trigger"=w270, "Voltage Scale"=w269, "Handle in"=w259) -> ("error out"=w271:errorcluster, "Handle_Out"=w272:u32)  [unwired: 1 in]
                n120 = call "Alazar_ChannelConfig - ATS-SDK.vi"("error in (no error)"=w271, "V scale"=w273, "Channel"=w260, "Handle in"=w272) -> ("error out"=w274:errorcluster, "Handle_Out"=w275:u32)  [unwired: 1 in, 1 out]
                n121 = call "AlazarStartCapture.vi"("Handle"=w275, "error in (no error)"=w274) -> ()  [unwired: 3 out]
              }
            }
            n122 = Unbundle By Name(w164) -> ("Y Scale Offset"=w165:dbl)
            n123 = Unbundle By Name(w161) -> ("rf points per line"=w167:i32, "lines per plane"=w166:i32)
            n124 = Divide(x=w167, y=2) -> (x/y=w170:dbl)
            n125 = call "PreCalcSecDisplayParams.vi"("delay mm"=w165, "pixels in y"=w170, "Background Value"=-100.0 ("element"), "Digitizer Settings"=w161, "pixels in x"=w166) -> ("Cluster out"=w172:T29)  [unwired: 6 in]
          }
          frame #1 {
            # "save eye if selected"
            # "Get data and feed to other loop"
            n126 = Unbundle By Name(w285) -> ("bits A/D"=w288:i8, "Samp Rate (Hz)"=w289:dbl)
            n127 = Unbundle By Name(w287) -> ("DataBufferQ"=w301:refnum<queue>, "Stop"=w300:refnum<notifier>)
            n128 = expression code="x*1E-6"(w289) -> (w307:dbl)
            n129 = while {
              tunnel: w304 -> [w337]
              tunnel: [w334] -> w308
              tunnel: w294 -> [w336]
              tunnel: w306 -> [w335]
              tunnel: w303 -> [w332]
              tunnel: w307 -> [w331]
              tunnel: [w330] -> w305
              shift-right: [w328] -> _
              shift-left: _ -> [w329]
              tunnel: w287 -> [w327]
              tunnel: w298 -> [w325]
              tunnel: w299 -> [w324]
              tunnel: w296 -> [w323]
              tunnel: w295 -> [w322]
              tunnel: w293 -> [w318]
              tunnel: w288 -> [w317]
              tunnel: w286 -> [w315]
              tunnel: w283 -> [w314]
              tunnel: w285 -> [w316]
              tunnel: w284 -> [w313]
              i -> [w338]
              stop <- w334 stop-if-true
              n130 = local read "append letter"() -> (w326:i8)
              n131 = local read "File Name"() -> (w320:string)
              n132 = event shown="[5] \"Gain\": Value Change" {
                selector: _ -> [_ _ _ _ _ _ _ _ _ _ _ _ _ _ _ _ _ _ _ _]
                dyn-events: _ -> [_ _ _ _ _ _ _ _ _ _ _ _ _ _ _ _ _ _ _ _]
                timeout: 40 -> [_ _ _ _ _ _ _ _ _ _ _ _ _ _ _ _ _ _ _ _]
                tunnel: w338 -> [w356 _ _ _ _ _ _ _ _ _ _ _ _ _ _ _ _ _ _ _]
                tunnel: w337 -> [_ w461 _ _ _ _ _ _ _ _ _ _ _ _ _ _ _ _ _ _]
                tunnel: [_ _ _ w501 TRUE TRUE TRUE _ _ _ _ _ _ _ _ _ _ _ _ _] -> w334
                tunnel: w320 -> [w355 _ _ _ _ _ _ _ _ _ _ _ _ _ w572 _ _ _ w637 _]
                tunnel: w336 -> [_ _ _ _ _ _ _ w524 _ _ _ _ _ _ _ _ _ _ _ _]
                tunnel: w335 -> [w354 _ _ _ _ _ _ _ _ _ _ _ _ _ _ _ _ _ _ _]
                tunnel: w332 -> [w353 w460 _ _ _ _ _ _ _ _ _ _ _ _ _ w587 _ _ _ _]
                tunnel: w331 -> [w352 _ _ _ _ _ _ _ _ _ _ _ _ _ _ _ _ _ _ _]
                tunnel: [_ _ _ w501 _ _ _ _ _ _ _ _ _ _ _ _ _ _ _ _] -> w330
                tunnel: w329 -> [w346 _ _ _ _ _ _ _ _ _ _ _ _ _ _ _ _ _ _ _]
                tunnel: [w345 _ _ _ _ _ _ _ _ _ _ _ _ _ _ _ _ _ _ _] -> w328
                tunnel: w327 -> [w351 _ _ w499 w503 w511 w515 _ _ _ _ _ _ _ w581 _ _ w627 w635 _]
                tunnel: w326 -> [w344 _ _ _ _ _ _ _ _ _ _ _ _ w564 w573 _ _ _ w636 _]
                tunnel: w325 -> [_ _ _ _ _ _ _ _ _ _ _ _ _ _ _ w591 w623 _ _ _]
                tunnel: w324 -> [_ _ _ _ _ _ _ _ _ _ _ _ _ _ _ w590 _ _ _ _]
                tunnel: w323 -> [w350 _ _ _ _ _ _ _ _ _ _ _ _ _ w567 _ _ _ w630 _]
                tunnel: w322 -> [_ _ w491 _ _ _ _ _ _ _ _ _ _ _ _ _ _ _ _ _]
                tunnel: T18 {"DataBufferQ"=refnum, "LastNQ"=refnum, "LastNBMPQ"=refnum, "SaveRawN"=refnum, "StopN"=refnum} ("Qs and Notis") -> [_ _ _ _ _ _ _ _ _ _ _ _ _ _ w577 _ _ _ w633 _]
                tunnel: "Sector?" -> [w343 w459 _ _ _ _ _ _ _ _ _ _ _ _ _ w585 _ _ _ _]
                tunnel: w318 -> [_ _ _ _ _ _ _ _ _ _ _ _ _ _ _ _ _ _ _ w649]
                tunnel: w317 -> [w342 _ _ _ _ _ _ _ _ _ _ _ _ _ w570 _ _ _ w629 _]
                tunnel: w316 -> [w340 _ _ _ _ _ w518 _ _ _ _ _ _ _ w568 w582 _ _ w628 _]
                tunnel: w315 -> [w341 _ _ _ _ _ _ _ _ _ _ _ _ _ w569 _ _ _ _ w648]
                tunnel: w314 -> [_ _ _ _ _ _ w519 _ _ _ _ _ _ _ _ _ _ _ _ _]
                tunnel: w313 -> [w339 _ _ _ _ _ _ _ _ _ _ _ _ _ _ _ _ _ _ _]
                event Timeout {
                  n133 = event-data() -> ()  [unwired: 1 in, 2 out]
                  n134 = Unbundle By Name(w351) -> ("DataBufferQ"=w349:refnum<queue>)
                  n135 = Dequeue Element(queue=w349) -> (element=w348:T11)  [unwired: 2 in, 3 out]
                  n136 = Unbundle(w348) -> (w347:bool)  [unwired: 4 out]
                  "No data\nEntering\nQueue" <- w347
                  n137 = case shown="False" w347 {
                    tunnel: w356 -> [w374 _]
                    tunnel: w355 -> [w373 _]
                    tunnel: w354 -> [w372 _]
                    tunnel: w353 -> [w371 _]
                    tunnel: w352 -> [w370 _]
                    tunnel: w351 -> [w369 _]
                    tunnel: w350 -> [w368 _]
                    tunnel: w348 -> [w366 _]
                    tunnel: w346 -> [w365 w457]
                    tunnel: [w364 w457] -> w345
                    tunnel: w344 -> [w362 _]
                    tunnel: w343 -> [w361 _]
                    tunnel: w342 -> [w360 _]
                    tunnel: w341 -> [w359 _]
                    tunnel: w340 -> [w358 _]
                    tunnel: w339 -> [w357 _]
                    frame False {
                      n138 = stacked-sequence {
                        tunnel: w374 -> [w401 w440]
                        tunnel: w373 -> [_ w430]
                        tunnel: w372 -> [w399 _]
                        tunnel: w371 -> [w396 _]
                        tunnel: w370 -> [w395 _]
                        tunnel: w369 -> [w389 w438]
                        tunnel: w368 -> [_ w433]
                        tunnel: "Save Raw" -> [_ w435]
                        tunnel: w366 -> [w392 w434]
                        tunnel: w365 -> [w381 _]
                        tunnel: [w379 _] -> w364
                        tunnel: "Pause" -> [w378 w432]
                        tunnel: w362 -> [_ w428]
                        tunnel: w361 -> [w377 _]
                        tunnel: w360 -> [w376 w426]
                        tunnel: w359 -> [_ w425]
                        tunnel: w358 -> [_ w424]
                        tunnel: w357 -> [_ _]
                        frame #0 {
                          # "set scale after first image"
                          # "Get and display data"
                          n139 = Unbundle(w392) -> ("gain"=w388:dbl, "wfm"=w387:i16[][])  [unwired: 3 out]
                          n140 = Increment(x=w401) -> (x+1=→"Current Image":i32)
                          n141 = call "SubMean.vi"("Bit Depth"=w376, "Scan Data In"=w387, "Samp Rate (MHz)"=w395, "Filter Prams"="Filter Prams", "Type of Mean"="Type of Mean") -> ("Array"=w400:dbl[][])  [unwired: 1 in, 2 out]
                          n142 = Unbundle By Name(w389) -> ("LastNQ"=w391:refnum<queue>)
                          n143 = case shown="False" w377 {
                            tunnel: [w412 w421] -> w397
                            tunnel: w400 -> [w411 w422]
                            tunnel: w399 -> [w410 w423]
                            tunnel: w396 -> [_ w420]
                            frame False {
                              # "Linear array data"
                              n144 = for {
                                tunnel: [w415] -> w412 mode=indexing
                                tunnel: w411 -> [w414] mode=indexing
                                tunnel: w410 -> [w413]
                                n145 = for {
                                tunnel: [w419] -> w415 mode=indexing
                                tunnel: w414 -> [w418] mode=indexing
                                tunnel: w413 -> [w416]
                                n146 = Absolute Value(x=w418) -> (abs(x)=w417:dbl)
                                n147 = Index Array(array=w416, index=w417) -> (element=w419:sgl)
                                }
                              }
                            }
                            frame True {
                              # "Convert to sector"
                              n148 = call "AvisoSectorConvert.vi"("output cluster"=w420, "Log Lookup"=w423, "Raw In"=w422) -> ("Sector out"=w421:dbl[][])  [unwired: 8 in]
                            }
                          }
                          n149 = Bundle("gain"=w388, "wfm"=w387) -> (w386:cluster{"gain":dbl, "wfm":i16[][]})  [unwired: 1 in]
                          n150 = case shown="True" w378 {
                            tunnel: w391 -> [w404 w407]
                            tunnel: [w404 w406] -> w390
                            tunnel: w386 -> [_ w405]
                            frame False {
                            }
                            frame True {
                              n151 = Lossy Enqueue Element(queue=w407, element=w405) -> (queue out=w406:refnum<queue>)  [unwired: 1 in, 3 out]
                            }
                          }
                          n152 = Get Queue Status(queue=w390) -> (# elements in queue=w375:i32)  [unwired: 2 in, 7 out]
                          "In Queue" <- w375
                          "queue bar" <- w375
                          n153 = case shown="2" w375 {
                            frame 0, Default {
                            }
                            frame 2 {
                              n154 = stacked-sequence {
                                frame #0 {
                                n155 = local read "distance?"() -> (w402:bool)
                                n156 = property on="distance?" class="Bool (strict)"("Val(Sgnl)"=w402) -> ()  [unwired: 2 in, 2 out]
                                }
                                frame #1 {
                                n157 = property on="1:1\nAspect" class="Bool (strict)"("Val(Sgnl)"=FALSE ("Value (Signaling)")) -> ()  [unwired: 2 in, 2 out]
                                }
                              }
                            }
                          }
                          n158 = flat-sequence {
                            tunnel: w397 -> [w408]
                            tunnel: [w409] -> w379
                            frame #0 {
                              "Raw data" <- w408
                            }
                            frame #1 {
                              n159 = Tick Count (ms)() -> (millisecond timer value=w409:u32)
                            }
                          }
                          n160 = Subtract(x=w379, y=w381) -> (x-y=w385:u32)
                          n161 = To Double Precision Float(number=w385) -> (double precision float=w384:dbl)
                          n162 = expression code="1000/x"(w384) -> (w383:dbl)
                          n163 = call <vilib>:"Mean PtByPt.vi"("x"=w383, "sample length"=10) -> ("mean"=→"fps":dbl)  [unwired: 2 in, 1 out]
                        }
                        frame #1 {
                          w427 = "_" ("string")
                          # "Save jpg if selected"
                          n164 = Type Cast(x=w428) -> (*(type *) &x=w431:string)  [unwired: 1 in]
                          n165 = invoke on="Raw data" class="IntGraph (strict)" method="Get Image"("image depth"=24) -> ("image data"=w436:T13)  [unwired: 5 in, 5 out]
                          n166 = Concatenate Strings(w430, w427, w431, w427) -> (w429:string)
                          n167 = case shown="True" w435 {
                            tunnel: w440 -> [_ w448]
                            tunnel: w429 -> [_ w451]
                            tunnel: w436 -> [_ w453]
                            tunnel: w434 -> [_ w452]
                            tunnel: w433 -> [_ w447]
                            tunnel: w426 -> [_ w446]
                            tunnel: w425 -> [_ w445]
                            tunnel: w424 -> [_ w444]
                            frame False {
                            }
                            frame True {
                              n168 = Unbundle(w452) -> ("gain"=w450:dbl, "wfm"=w449:i16[][])  [unwired: 3 out]
                              n169 = case shown="True" FALSE {
                                tunnel: w453 -> [_ w456]
                                tunnel: w451 -> [_ w455]
                                tunnel: w448 -> [_ w454]
                                frame False {
                                }
                                frame True {
                                n170 = call "RT_Save_JPG.vi"("Movie Name"=w455, "Frame"=w454, "image data"=w456) -> ()  [unwired: 9 in]
                                }
                              }
                              n171 = call "RT_Save_EYE.vi"("Motion Settings"=w445, "Digitizer Gain"=w450, "bits A/D"=w446, "Eye Name"=w451, "Digitizer Settings"=w444, "Scan Info"=w447, "Frame"=w448, "Data"=w449) -> ()  [unwired: 4 in]
                            }
                          }
                          n172 = Unbundle By Name(w438) -> ("LastN_JPG_Q"=w437:refnum<queue>)
                          n173 = case shown="True" w432 {
                            tunnel: w437 -> [_ w442]
                            tunnel: w436 -> [_ w441]
                            frame False {
                            }
                            frame True {
                              n174 = Lossy Enqueue Element(queue=w442, element=w441) -> ()  [unwired: 1 in, 4 out]
                            }
                          }
                        }
                      }
                    }
                    frame True {
                      # "If time out or error in acquisition don't do anything"
                    }
                  }
                }
                event "distance?", "Sector?": Value Change {
                  w458 = u8 1 ("X Scale.Scale Fit")
                  # "Choose distance or index scales"
                  n175 = event-data() -> ()  [unwired: 1 in, 3 out]
                  n176 = case shown="True" "distance?" {
                    tunnel: [w468 w476] -> w466
                    tunnel: [w467 w475] -> w465
                    tunnel: [w468 w474] -> w464
                    tunnel: [w467 w473] -> w463
                    tunnel: w461 -> [_ w471]
                    tunnel: w459 -> [_ w469]
                    tunnel: w460 -> [_ w470]
                    frame False {
                      w467 = 1
                      w468 = 0
                    }
                    frame True {
                      n177 = Unbundle(w471) -> ("Y Scale Offset"=w480:dbl, "Y Scale Multi"=w479:dbl, "X Scale Offset"=w478:dbl, "X Scale Multi"=w477:dbl, "Gate Distance"=w472:dbl)
                      n178 = case shown="True" w469 {
                        tunnel: w480 -> [w482 w490]
                        tunnel: w479 -> [w481 _]
                        tunnel: w478 -> [w484 _]
                        tunnel: w477 -> [w483 _]
                        tunnel: [w484 0.0 ("X Scale.Offset and Multiplier:Offset")] -> w476
                        tunnel: [w483 w486] -> w475
                        tunnel: [w482 w490] -> w474
                        tunnel: [w481 w485] -> w473
                        tunnel: w472 -> [_ _]
                        tunnel: w470 -> [_ w487]
                        frame False {
                        }
                        frame True {
                          # "sector"
                          n179 = Unbundle(w487) -> ("scales"=w488:cluster{"inc x (mm)":dbl, "inc y (mm)":dbl})  [unwired: 6 out]
                          n180 = Unbundle(w488) -> ("inc x (mm)"=w486:dbl, "inc y (mm)"=w485:dbl)
                        }
                      }
                    }
                  }
                  n181 = property on="Raw data" class="IntGraph (strict)"("X Scale.Offset and Multiplier:Offset"=w466, "X Scale.Offset and Multiplier:Multiplier"=w465, "Y Scale.Offset and Multiplier:Offset"=w464, "Y Scale.Offset and Multiplier:Multiplier"=w463, "XScale.ScaleFit"=w458, "YScale.ScaleFit"=w458) -> ()  [unwired: 2 in, 2 out]
                }
                event "LowTime", "Gate Length": Value Change {
                  n182 = event-data() -> ()  [unwired: 1 in, 6 out]
                  n183 = case shown="True" w491 {
                    frame False {
                      n184 = flat-sequence {
                        tunnel: refnum<k21> "QuantGate" ("task in") -> [w495]
                        tunnel: [w494] -> w493
                        tunnel: w493 -> [_]
                        frame #0 {
                          n185 = call <vilib>:"DAQmx Stop Task.vi"("task/channels in"=w495) -> ("task out"=w494:refnum<k21>)  [unwired: 13 in, 1 out]
                        }
                        frame #1 {
                          n186 = call "FrameSync.vi"("LowTime"="LowTime", "Gate Length"="Gate Length") -> ()  [unwired: 8 in, 2 out]
                        }
                      }
                    }
                    frame True {
                    }
                  }
                }
                event "stop": Value Change {
                  w501 = TRUE
                  n187 = event-data() -> ()  [unwired: 1 in, 2 out]
                  n188 = Unbundle By Name(w499) -> ("Stop"=w498:refnum<notifier>)
                  n189 = Send Notification(notification=TRUE, notifier=w498) -> ()  [unwired: 1 in, 2 out]
                }
                event "Acquisition Parameters.Sampling Rate", "Probe", "Bang Trig", "Software Gate", "c (m/s)", "Acquisition Parameters.Ref Delay (ms)", "Acquisition Parameters.rf points per line", "Acquisition Parameters.rf lines", "Acquisition Parameters.Dig Scale": Value Change {
                  # "restart loops if new probe selected"
                  # "Restart loops with new digitizer settings"
                  n190 = event-data() -> ()  [unwired: 1 in, 6 out]
                  n191 = Unbundle By Name(w503) -> ("Stop"=w502:refnum<notifier>)
                  n192 = Send Notification(notification=TRUE, notifier=w502) -> ()  [unwired: 1 in, 2 out]
                }
                event "Gain": Value Change {
                  # "Use this to force selected gain."
                  # "Restart loops with new gain setting"
                  n193 = event-data() -> ()  [unwired: 1 in, 6 out]
                  n194 = Unbundle By Name(w511) -> ("Stop"=w510:refnum<notifier>)
                  n195 = Send Notification(notification=TRUE, notifier=w510) -> ()  [unwired: 1 in, 2 out]
                  n196 = local write "Overide Gain?"(TRUE ("Overide Gain?")) -> ()
                  n197 = property on="Acquisition Parameters" class="Clust (strict)"() -> ("Value"=w509:T1)  [unwired: 2 in, 2 out]
                  n198 = Bundle By Name(cluster=w509, "Dig Scale"="Gain") -> (w508:T1)
                  n199 = property on="Acquisition Parameters" class="Clust (strict)"("Value"=w508) -> ()  [unwired: 2 in, 2 out]
                }
                event "SetDig": Value Change {
                  n200 = event-data() -> ()  [unwired: 1 in, 1 out]
                  n201 = Unbundle By Name(w515) -> ("Stop"=w516:refnum<notifier>)
                  n202 = Send Notification(notification=TRUE, notifier=w516) -> ()  [unwired: 1 in, 2 out]
                  n203 = call "SetUpDigi.vi"("Digitizer Settings"=w518, "Motion Settings In"=w519) -> ()  [unwired: 11 in, 7 out]
                }
                event "Patient Info": Value Change {
                  n204 = event-data() -> ()  [unwired: 1 in, 2 out]
                  n205 = call "Info.vi"("Patient Info In"=w524) -> ("NewCase?"=w520:bool, "FileName"=→"File Name":string, "Patient Info Out"=w525:T30)  [unwired: 8 in]
                  n206 = property on="Patient Info" class="Bool (strict)"("Value"=FALSE ("Patient Info")) -> ()  [unwired: 2 in, 2 out]
                  n207 = Unbundle By Name(w525) -> ("Plane"=w523:i8)
                  n208 = case shown="True" w520 {
                    frame False {
                    }
                    frame True {
                      # "Rest Letter Index"
                      n209 = local write "append letter"(i8 65 ("append letter")) -> ()
                    }
                  }
                  n210 = local write "Plane"(w523) -> ()
                }
                event "Plane": Mouse Up; "Scan Location": Value Change {
                  n211 = event-data() -> ()  [unwired: 1 in, 4 out]
                  n212 = global read "PatientGlobals.vi" "Patient Info"() -> (w527:T30)
                  n213 = Bundle By Name(cluster=w527, "Plane"="Plane", "Scan Location"="Scan Location") -> (w528:T30)
                  n214 = global write "PatientGlobals.vi" "Patient Info"(w528) -> ()
                }
                event "dB Range": Value Change {
                  n215 = event-data() -> ("NewVal"=w531:cluster{i32, i32})  [unwired: 1 in, 5 out]
                  n216 = Unbundle(w531) -> (w533:i32, w534:i32)
                  n217 = property on="Raw data" class="IntGraph (strict)"() -> ("ZScale.Range"=w532:T31)  [unwired: 2 in, 2 out]
                  n218 = Bundle By Name(cluster=w532, "Minimum"=w534, "Maximum"=w533) -> (w535:T31)
                  n219 = property on="Raw data" class="IntGraph (strict)"("ZScale.Range"=w535) -> ()  [unwired: 2 in, 2 out]
                }
                event "Visible": Value Change {
                  n220 = event-data() -> ("NewVal"=w536:bool)  [unwired: 1 in, 5 out]
                  n221 = property on="Raw data" class="IntGraph (strict)"("Active Cursor"=u32 0, "Cursor.Visible"=w536, "Active Cursor"=u32 1, "Cursor.Visible"=w536) -> ()  [unwired: 2 in, 2 out]
                }
                event "Center": Value Change {
                  n222 = event-data() -> ()  [unwired: 1 in, 6 out]
                  n223 = property on="Raw data" class="IntGraph (strict)"() -> ("XScale.Maximum"=w539:dbl, "XScale.Minimum"=w540:dbl, "YScale.Maximum"=w541:dbl, "YScale.Minimum"=w542:dbl)  [unwired: 2 in, 2 out]
                  n224 = Add(x=w539, y=w540) -> (x+y=w543:dbl)
                  n225 = Add(x=w541, y=w542) -> (x+y=w544:dbl)
                  n226 = expression code="x/2"(w543) -> (w545:dbl)
                  n227 = expression code="x/2"(w544) -> (w546:dbl)
                  n228 = Bundle(w545, w546) -> (w549:cluster{dbl, dbl})  [unwired: 1 in]
                  n229 = property on="Raw data" class="IntGraph (strict)"("Active Cursor"=u32 0, "Cursor.Cursor Position"=w549, "Active Cursor"=u32 1, "Cursor.Cursor Position"=w549) -> ()  [unwired: 2 in, 2 out]
                }
                event "Raw data": Cursor Move {
                  n230 = event-data() -> ()  [unwired: 1 in, 1 out]
                  n231 = property on="Raw data" class="IntGraph (strict)"("Active Cursor"=u32 0, "Active Cursor"=u32 1) -> ("Cursor.Cursor Position"=w559:T32, "Cursor.Cursor Position"=w554:T32)  [unwired: 2 in, 2 out]
                  n232 = Subtract(x=w559, y=w554) -> (x-y=w555:T32)
                  n233 = Unbundle(w555) -> ("Cursor X"=w556:dbl, "Cursor Y"=w550:dbl)
                  n234 = Re/Im To Polar(2:w550, 3:w556) -> (1:w551:dbl)  [unwired: 1 out]
                  n235 = Number To Fractional String(number=w551, precision (6)=i16 2) -> (F-format string=w560:string)  [unwired: 2 in]
                  n236 = Concatenate Strings(w560, " mm") -> (w562:string)
                  n237 = property on="Raw data" class="IntGraph (strict)"("Active Cursor"=u32 0, "Cursor.Cursor Name"=w562) -> ()  [unwired: 2 in, 2 out]
                }
                event "Save Raw": Value Change {
                  n238 = event-data() -> ("NewVal"=w563:bool)  [unwired: 1 in, 5 out]
                  n239 = case shown="False" w563 {
                    tunnel: w564 -> [w565 _]
                    frame False {
                      n240 = Increment(x=w565) -> (x+1=w566:i8)
                      n241 = local write "append letter"(w566) -> ()
                    }
                    frame True {
                    }
                  }
                }
                event "Save All Queue": Value Change {
                  w580 = i16 1
                  # "Save last N files in queue"
                  n242 = event-data() -> ()  [unwired: 1 in, 2 out]
                  n243 = Unbundle By Name(w581) -> ("LastNQ"=w576:refnum<queue>, "LastN_JPG_Q"=w575:refnum<queue>)
                  n244 = Bundle(cluster=w577, "LastNQ"=w576, "LastNBMPQ"=w575) -> (w574:T18)  [unwired: 3 in]
                  n245 = Bundle(w580, w580, "N to save"="N to save") -> (w578:cluster{i16, i16, "N to save":u8})  [unwired: 1 in]
                  n246 = call "SaveQueueN.vi"("Digitizer Settings"=w568, "Motion Settings"=w569, "File Name"=w572, "Scan Info"=w567, "bits A/D"=w570, "append letter"=w573, "Qs and Notis"=w574, "Slider Indexes"=w578) -> ("append letter out"=w571:i8)  [unwired: 3 in]
                  n247 = local write "append letter"(w571) -> ()
                }
                event "1:1\nAspect": Value Change {
                  w584 = u8 1 ("X Scale.Scale Fit")
                  n248 = event-data() -> ()  [unwired: 1 in, 2 out]
                  n249 = case shown="False" w585 {
                    tunnel: [w603 w606] -> w589
                    tunnel: [w604 w607] -> w588
                    tunnel: w587 -> [_ w608]
                    tunnel: w582 -> [w605 _]
                    frame False {
                      n250 = Unbundle By Name(w605) -> ("lines per plane"=w604:i32, "rf points per line"=w603:i32)
                    }
                    frame True {
                      n251 = Unbundle(w608) -> ("pixels in x"=w607:i16, "pixels in y"=w606:i16)  [unwired: 5 out]
                    }
                  }
                  n252 = property on="Raw data" class="IntGraph (strict)"() -> ("X Scale.Offset and Multiplier:Multiplier"=w592:dbl, "Y Scale.Offset and Multiplier:Multiplier"=w593:dbl)  [unwired: 2 in, 2 out]
                  n253 = Multiply(x=w588, y=w592) -> (x*y=w594:dbl)
                  n254 = Multiply(x=w593, y=w589) -> (x*y=w595:dbl)
                  n255 = Unbundle(w590) -> ("Width"=w600:u32, "Height"=w602:u32)
                  n256 = local write "1:1\nAspect"(FALSE ("1:1\nAspect")) -> ()
                  n257 = Divide(x=w600, y=w594) -> (x/y=w596:dbl)
                  n258 = Divide(x=w602, y=w595) -> (x/y=w597:dbl)
                  n259 = Divide(x=w596, y=w597) -> (x/y=w601:dbl)
                  n260 = Greater?(x=w601, y=1.0) -> (0:w598:bool)
                  n261 = case shown="False" w598 {
                    tunnel: w600 -> [_ w622]
                    tunnel: w601 -> [w615 w621]
                    tunnel: w602 -> [w614 _]
                    tunnel: w591 -> [w609 w620]
                    tunnel: [w610 w616] -> w583
                    frame False {
                      n262 = Unbundle By Name(w609) -> ("Top"=w613:i16)
                      n263 = Multiply(x=w614, y=w615) -> (x*y=w611:dbl)
                      n264 = Add(x=w613, y=w611) -> (x+y=w612:dbl)
                      n265 = Bundle By Name(cluster=w609, "Bottom"=w612) -> (w610:T9)
                    }
                    frame True {
                      n266 = Unbundle By Name(w620) -> ("Left"=w618:i16)
                      n267 = Divide(x=w622, y=w621) -> (x/y=w619:dbl)
                      n268 = Add(x=w618, y=w619) -> (x+y=w617:dbl)
                      n269 = Bundle By Name(cluster=w620, "Right"=w617) -> (w616:T9)
                    }
                  }
                  n270 = property on="Raw data" class="IntGraph (strict)"("Plot Bounds"=w583, "XScale.ScaleFit"=w584, "YScale.ScaleFit"=w584) -> ()  [unwired: 2 in, 2 out]
                }
                event "Fill\nSpace": Value Change {
                  w624 = u8 1 ("X Scale.Scale Fit")
                  n271 = event-data() -> ()  [unwired: 1 in, 6 out]
                  n272 = property on="Raw data" class="IntGraph (strict)"("Plot Bounds"=w623, "XScale.ScaleFit"=w624, "YScale.ScaleFit"=w624) -> ()  [unwired: 2 in, 2 out]
                }
                event "Flush Queue": Value Change {
                  n273 = event-data() -> ()  [unwired: 1 in, 6 out]
                  n274 = Unbundle By Name(w627) -> ("LastNQ"=w626:refnum<queue>, "LastN_JPG_Q"=w625:refnum<queue>)
                  n275 = Flush Queue(queue=w625) -> ()  [unwired: 1 in, 3 out]
                  n276 = Flush Queue(queue=w626) -> ()  [unwired: 1 in, 3 out]
                }
                event "View Queue": Value Change {
                  # "Save files baed on queue selection"
                  n277 = event-data() -> ()  [unwired: 1 in, 6 out]
                  n278 = Unbundle By Name(w635) -> ("LastNQ"=w632:refnum<queue>, "LastN_JPG_Q"=w631:refnum<queue>)
                  n279 = Bundle(cluster=w633, "LastNQ"=w632, "LastNBMPQ"=w631) -> (w634:T18)  [unwired: 3 in]
                  n280 = call "ViewQueue.vi"("Image queue"=w631) -> ("Slider Indexes"=w639:cluster{i16, i16, i16}, "Save?"=w638:bool)  [unwired: 3 in]
                  n281 = case shown="True" w638 {
                    tunnel: w636 -> [_ w647]
                    tunnel: w639 -> [_ w646]
                    tunnel: w637 -> [_ w645]
                    tunnel: w634 -> [_ w644]
                    tunnel: w629 -> [_ w643]
                    tunnel: w630 -> [_ w642]
                    tunnel: w628 -> [_ w640]
                    frame False {
                    }
                    frame True {
                      n282 = call "SaveQueueN.vi"("Digitizer Settings"=w640, "File Name"=w645, "Scan Info"=w642, "bits A/D"=w643, "append letter"=w647, "Qs and Notis"=w644, "Slider Indexes"=w646) -> ("append letter out"=w641:i8)  [unwired: 4 in]
                      n283 = local write "append letter"(w641) -> ()
                    }
                  }
                }
                event "Save Setting Profile": Value Change {
                  # "Add profile case but check that Custom settings is selected."
                  n284 = event-data() -> ()  [unwired: 1 in, 6 out]
                  n285 = property on="Probe" class="Ring (strict)"() -> ("Value"=w653:u16, "NumItems"=w651:u32)  [unwired: 2 in, 2 out]
                  n286 = Increment(x=w653) -> (x+1=w650:u16)
                  n287 = Equal?(x=w650, y=w651) -> (x = y?=w652:bool)
                  n288 = case shown="True" w652 {
                    tunnel: w650 -> [_ w657]
                    tunnel: w649 -> [_ w656]
                    tunnel: w648 -> [_ w655]
                    frame False {
                    }
                    frame True {
                      n289 = Unbundle By Name(w655) -> ("Distance between\nscan lines (um)"=w654:sgl)
                      n290 = local read "Acquisition Parameters"() -> (w664:T1)
                      n291 = local read "Filter Prams"() -> (w661:T2)
                      n292 = local read "Timeout (s)"() -> (w663:dbl)
                      n293 = local read "Scan Info"() -> (w660:T3)
                      n294 = local read "Sector?"() -> (w662:bool)
                      n295 = call "Prompt User for Input"() -> ("New Case Name"=w659:string)  [unwired: 17 in, 2 out]
                      n296 = Bundle("New Case Name"=w659, "Distance between\nscan lines (um)"=w654, "Acquisition Parameters"=w664, "Timeout (s)"=w663, "Sector?"=w662, "Filter Prams"=w661, "Scan Info"=w660) -> (w658:T33)  [unwired: 1 in]
                      n297 = call "ReadOrSaveCases.vi"("Location"=w656, "New Case"=w658, "Save(T)\\Read(F)"=TRUE ("Save(T)\\Read(F)")) -> ("Case List"=w665:string[])  [unwired: 7 in, 1 out]
                      n298 = property on="Probe" class="Ring (strict)"("Strings []"=w665, "Value"=w657) -> ()  [unwired: 2 in, 2 out]
                    }
                  }
                }
              }
            }
            n299 = while {
              tunnel: [w683] -> w309
              tunnel: w300 -> [w686]
              tunnel: w301 -> [w669]
              tunnel: w295 -> [w677]
              tunnel: w297 -> [w676]
              tunnel: [w669] -> _
              tunnel: w285 -> [w668]
              tunnel: w283 -> [w667]
              stop <- w683 stop-if-true
              n300 = call "SoftwareGate_Rapid Read.vi"("Timeout (s)"="Timeout (s)", "Channel"="0", "Digitizer Settings"=w668, "AlazarCluster"=w676, "Motion Settings"=w667, "Software Gate"=w677) -> ("gain"=w674:dbl, "Array"=w682:i16[][], "Reverse?"=w681:bool, "error out"=w679:errorcluster)  [unwired: 6 in]
              n301 = case shown="True" w681 {
                tunnel: w682 -> [w688 w689]
                tunnel: [w687 w689] -> w671
                frame False {
                  n302 = call "ReverseData.vi"("Array in"=w688) -> ("Array out"=w687:i16[][])
                }
                frame True {
                }
              }
              n303 = Unbundle By Name(w679) -> ("status"=w678:bool)
              n304 = Wait on Notification(notifier=w686, timeout in ms (-1)=5) -> (timed out?=w684:bool)  [unwired: 2 in, 3 out]
              n305 = Not(x=w684) -> (.not. x?=w683:bool)
              n306 = Bundle("gain"=w674, "status"=FALSE, "Array"=w671, "timeout in ms (-1)"=0, "status"=w678) -> (w673:T34)  [unwired: 1 out]
              n307 = Lossy Enqueue Element(queue=w669, element=w673) -> ()  [unwired: 1 in, 4 out]
            }
            n308 = And(x=w309, y=w308) -> (x .and. y?=w302:bool)
            n309 = Unbundle By Name(w287) -> ("DataBufferQ"=w292:refnum<queue>, "LastNQ"=w291:refnum<queue>, "LastN_JPG_Q"=w290:refnum<queue>)
            n310 = case shown="True" w302 {
              tunnel: w292 -> [_ w312]
              tunnel: w291 -> [_ w311]
              tunnel: w290 -> [_ w310]
              frame False {
              }
              frame True {
                # "wipe buffers"
                n311 = Flush Queue(queue=w312) -> ()  [unwired: 1 in, 3 out]
                n312 = Flush Queue(queue=w311) -> ()  [unwired: 1 in, 3 out]
                n313 = Flush Queue(queue=w310) -> ()  [unwired: 1 in, 3 out]
              }
            }
          }
          frame #2 {
            n314 = case shown="\"AlazarTech\"" w691 {
              tunnel: w692 -> [_ _ w698]
              tunnel: w690 -> [_ w693 w697]
              frame "Acqiris Digitizer", Default {
              }
              frame "NI Digitizer" {
                n315 = Unbundle By Name(w693) -> ("Digitizer ID Cluster.NI Instr Handles"=w695:refnum<k15>[])
                n316 = Index Array(array=w695) -> (element=w694:refnum<k15>)  [unwired: 1 in]
                n317 = call <instrlib>:"niScope Abort.vi"("instrument handle"=w694) -> ()  [unwired: 13 in, 2 out]
              }
              frame "AlazarTech" {
                n318 = Unbundle By Name(w697) -> ("Digitizer ID Cluster.Acqiris/Alazar/SP ID"=w696:u32[])
                n319 = Unbundle By Name(w698) -> ("data value reference"=w699:refnum<data-value>)
                n320 = for {
                  tunnel: w696 -> [w700] mode=indexing
                  n321 = call "AlazarAbortAsyncRead.vi"("Handle"=w700) -> ()  [unwired: 1 in, 3 out]
                }
                n322 = Delete Data Value Reference(data value reference=w699) -> ()  [unwired: 1 in, 2 out]
              }
            }
          }
        }
      }
    }
    frame #3 {
      w703 = TRUE ("force destroy? (F)")
      n323 = Unbundle By Name(w701) -> ("DataBufferQ"=w707:refnum<queue>, "LastNQ"=w705:refnum<queue>, "LastN_JPG_Q"=w704:refnum<queue>, "Stop"=w706:refnum<notifier>)
      n324 = Release Queue(queue=w704, force destroy? (F)=w703) -> ()  [unwired: 1 in, 3 out]
      n325 = Release Notifier(notifier=w706, force destroy? (F)=w703) -> ()  [unwired: 1 in, 3 out]
      n326 = Release Queue(queue=w707, force destroy? (F)=w703) -> ()  [unwired: 1 in, 3 out]
      n327 = Release Queue(queue=w705, force destroy? (F)=w703) -> ()  [unwired: 1 in, 3 out]
      n328 = case shown="\"NI Digitizer\"" w708 {
        tunnel: w702 -> [_ w712]
        frame "Acqiris Digitizer", Default {
        }
        frame "NI Digitizer" {
          n329 = Unbundle By Name(w712) -> ("Digitizer ID Cluster.NI Instr Handles"=w711:refnum<k15>[])
          n330 = Index Array(array=w711) -> (element=w710:refnum<k15>)  [unwired: 1 in]
          n331 = call <instrlib>:"niScope Close.vi"("instrument handle"=w710) -> ()  [unwired: 1 in, 14 out]
        }
      }
      n332 = local write "stop"(FALSE ("stop out")) -> ()
    }
  }
  n333 = global write "DigitizerGlobals.vi" "Digitizer Settings"(w2) -> ()
